vi "Continuous Serial Write and Read 1kHz.vi"() -> ()   [LabVIEW 2017]
doc: "This example performs writes and reads on a serial port, as directed by the user. You can press the Write and Read buttons, and change the Read Count, while the example is running.\n\nThe parameters set for the serial port must match the parameters of the connected instrument or device. In this example, the Read Count parameter specifies the number of bytes that the serial port reads. If there were more bytes at the port than the specified number, those bytes would not be read. If there were less bytes at the port than the specified number, you would receive a timeout error.\n\nThis example expands upon the flow control options for XON and XOFF, allowing the user to choose those control characters. Also, the user can enable or disable a termination character. Some devices require a termination character in order to identify the end of command strings. Some devices send a termination character to signify the end of data to be read. This example shows how you can end the Read operation once a termination character is detected in the buffer and/or append a termination character at the end of the Write data."
uses:
  C:/Program Files (x86)/National Instruments/LabVIEW 2017/examples/Instrument IO/Serial/support/Serial - Settings.ctl
  C:/Program Files (x86)/National Instruments/LabVIEW 2017/examples/Instrument IO/Serial/support/Serial - XON-XOFF Characters.ctl
  C:/Program Files (x86)/National Instruments/LabVIEW 2017/examples/Instrument IO/Serial/support/Serial - ASCII Characters.ctl
  <vilib>/Platform/TimedLoop/XDataNode/timing_clust.ctl
  <vilib>/Platform/TimedLoop/XDataNode/nitl_modes.ctl
  <vilib>/Platform/TimedLoop/XDataNode/wakeup.ctl
  <vilib>/Instr/_visa.llb/VISA Configure Serial Port (Instr).vi
  <vilib>/platform/TimedLoop/XDataNode/XDataNode.xnode
  <vilib>/Platform/TimedLoop/XDataNode/XDNodeRunTimeDep.lvlib
panel:
  in  "Termination Character":u8=10 format="%.0x"
  in  "End Write on Termination Character?":bool=TRUE
  in  "Stop":bool
  in  "Read Count":u32=1000
  out "Response":string="\r\n\r\n\r\n\r\n0.01 0.01 0.01 0.00\r\n0.00 0.00 0.01 0.00\r\n0.00 0.01 0.00 0.00\r\n0.01 0.00 0.01 0.00\r\n0.00 0.01 0.00 0.00\r\n0.01 0.00 0.00 0.00\r\n0.01 0.01 0.01 0.00\r\n0.01 -0.00 -0.00 0.00\r\n0.01 0.01 0.01 0.00\r\n0.01 0.01 0.01 0.00\r\n0.01 0.00 -0.00 0.00\r\n0.00 0.01 0.01 0.00\r\n0.01 0.01 0.00 0.00\r\n0.01 0.01 0.01 0.00\r\n0.00 0.00 0.00 0.00\r\n0.01 0.01 0.01 0.00\r\n0.01 0.00 0.00 0.00\r\n0.00 0.01 0.01 0.00\r\n0.01 0.01 0.01 0.00\r\n0.01 0.01 0.01 0.00\r\n0.01 0.01 0.01 0.00\r\n0.01 0.00 0.01 0.00\r\n0.01 0.00 0.01 0.00\r\n0.01 0.00 0.01 0.00\r\n0.01 0.01 0.01 0.00\r\n0.01 0.00 0.00 0.00\r\n0.00 0.01 0.01 0.00\r\n-0.00 0.01 0.01 0.00\r\n0.00 0.00 0.01 0.00\r\n0.01 0.01 0.01 0.00\r\n0.00 0.01 0.01 0.00\r\n0.01 0.01 0.01 0.00\r\n0.00 0.01 0.01 0.00\r\n0.00 0.01 0.01 0.00\r\n0.01 0.00 0.01 0.00\r\n0.01 0.00 0.00 0.00\r\n0.01 0.01 0.01 0.00\r\n0.00 0.01 0.00 0.00\r\n0.01 0.01 0.01 0.00\r\n0.00 0.01 0.00 0.00\r\n0.01 0.01 0.01 0.00\r\n0.01 0.01 0.01 0.00\r\n0.00 0.01 0.01 0.00\r\n0.01 0.00 0.01 0.00\r\n0.01 0.01 0.01 0.00\r\n0.01 0.01 0.01 0.00\r\n0.00 0.00 0.01 0.00\r\n0.00 -0.00 0.00 0.00\r\n0.01 0.01 0.00 0.00\r\n0.01 0.01 0.01 0.00\r\n0.01 0.00 0.00 0.00\r\n0.01 0.01 0.01 0.00\r\n0.01 0.01 0.00 0.00\r\n0.01 0.01 0.00 0.00\r\n0.01 0.01 0.01 0.00\r\n0.01 0.00 0.01 0.00\r\n0.00 0.01 0.01 0.00\r\n0.01 0.01 0.01 0.00\r\n0.00 0.01 0.01 0.00\r\n0.01 0.00 0.01 0.00\r\n0.01 0.00 0.01 0.00\r\n0.01 0.01 0.01 0.00\r\n0.00 0.01 0.01 0.00\r\n0.01 0.00 0.01 0.00\r\n0.00 0.01 0.00 0.00\r\n0.01 0.01 0.01 0.00\r\n0.00 0.00 0.00 0.00\r\n0.00 0.01 0.00 0.00\r\n0.01 0.00 0.01 0.00\r\n0.01 0.01 0.00 0.00\r\n0.00 0.01 0.00 0.00\r\n0.01 0.01 0.00 0.00\r\n0.01 0.01 0.01 0.00\r\n0.01 0.01 0.01 0.00\r\n0.01 0.01 0.01 0.00\r\n0.01 0.01 0.00 0.00\r\n0.01 0.01 0.01 0.00\r\n0.01 0.00 0.01 0.00\r\n0.00 0.01 0.01 0.00\r\n-0.00 0.01 0.01 0.00\r\n0.00 0.01 0.01 0.00\r\n0.00 -0.00 0.00 0.00\r\n0.01 0.01 0.01 0.00\r\n0.01 0.01 0.00 0.00\r\n0.01 0.01 0.01 0.00\r\n0.00 0.01 0.01 0.00\r\n0.01 0.00 0.01 0.00\r\n0.01 0.00 0.00 0.00\r\n0.01 0.01 0.01 0.00\r\n0.01 0.01 0.01 0.00\r\n0.00 0.01 0.00 0.00\r\n0.01 0.01 0.01 0.00\r\n0.01 0.01 0.00 0.00\r\n0.01 0.00 -0.00 0.00\r\n0.01 0.01 0.01 0.00\r\n0.00 0.00 0.01 0.00\r\n0.00 0.00 0.00 0.00\r\n0.01 0.01 0.01 0.00\r\n0.01 0.01 0.01 0.00\r\n0.01 0.01 0.01 0.00\r\n0.01 0.01 0.01 0.00\r\n0.01 0.01 0.01 0.00\r\n0.01 0.01 0.01 0.00\r\n0.01 0.01 0.01 0.00\r\n0.01 0.01 0.01 0.00\r\n0.01 0.01 0.01 0.00\r\n0.00 0.01 0.01 0.00\r\n0.01 0.01 0.00 0.00\r\n0.01 0.01 0.00 0.00\r\n0.00 0.01 0.01 0.00\r\n0.01 0.01 0.00 0.00\r\n0.01 0.01 0.01 0.00\r\n0.00 0.01 0.01 0.00\r\n0.01 0.02 0.01 0.00\r\n0.01 0.01 0.01 0.00\r\n0.01 0.00 0.00 0.00\r\n0.00 0.01 0.01 0.00\r\n0.01 0.02 0.01 0.00\r\n0.01 0.01 0.01 0.00\r\n0.01 0.01 0.01 0.00\r\n0.01 0.00 0.01 0.00\r\n0.01 0.01 0.01 0.00\r\n0.01 0.01 0.01 0.00\r\n0.00 0.00 0.01 0.00\r\n0.01 0.00 0.00 0.00\r\n0.00 0.00 0.01 0.00\r\n0.01 0.01 0.01 0.00\r\n0.01 0.01 0.00 0.00\r\n0.00 0.01 0.01 0.00\r\n0.01 0.00 0.01 0.00\r\n0.01 0.00 0.01 0.00\r\n0.01 0.01 0.01 0.00\r\n0.01 0.01 0.01 0.00\r\n0.00 0.00 0.00 0.00\r\n0.01 0.01 0.01 0.00\r\n0.00 0.01 0.01 0.00\r\n0.01 0.00 0.00 0.00\r\n0.00 0.01 0.00 0.00\r\n0.01 0.01 0.02 0.00\r\n0.00 0.01 0.01 0.00\r\n0.00 0.01 0.01 0.00\r\n0.01 0.01 0.01 0.00\r\n0.01 0.00 0.01 0.00\r\n0.01 0.01 0.01 0.00\r\n0.01 0.01 0.01 0.00\r\n0.01 0.01 0.01 0.00\r\n0.01 0.01 0.01 0.00\r\n0.01 0.01 0.01 0.00\r\n0.00 0.01 0.01 0.00\r\n0.00 0.01 0.01 0.00\r\n0.01 0.01 0.01 0.00\r\n0.01 0.01 0.01 0.00\r\n0.01 0.00 0.01 0.00\r\n0.01 0.01 0.01 0.00\r\n0.01 0.01 0.01 0.00\r\n0.01 0.01 0.01 0.00\r\n0.01 0.01 0.01 0.00\r\n0.01 0.01 0.02 0.00\r\n0.01 0.01 0.01 0.00\r\n0.00 0.00 0.01 0.00\r\n0.01 0.01 0.01 0.00\r\n0.00 0.01 0.01 0.00\r\n0.01 0.01 0.01 0.00\r\n0.00 0.01 0.01 0.00\r\n0.00 0.01 0.01 0.00\r\n0.00 0.01 0.01 0.00\r\n0.01 0.00 0.01 0.00\r\n0.01 0.01 0.01 0.00\r\n0.01 0.01 0.01 0.00\r\n0.01 0.00 0.01 0.00\r\n0.01 0.01 0.01 0.00\r\n0.01 0.01 0.01 0.00\r\n0.01 0.01 0.01 0.00\r\n0.01 0.00 0.00 0.00\r\n0.01 0.01 0.01 0.00\r\n0.01 0.01 0.01 0.00\r\n0.01 -0.00 0.00 0.00\r\n0.00 0.01 0.01 0.00\r\n0.01 0.01 0.01 0.00\r\n0.01 0.01 0.00 0.00\r\n0.00 0.00 0.00 0.00\r\n0.01 0.00 0.00 0.00\r\n0.01 0.00 0.00 0.00\r\n0.00 0.01 0.01 0.00\r\n0.01 0.01 0.01 0.00\r\n0.01 0.01 0.01 0.00\r\n0.01 0.01 0.01 0.00\r\n0.00 0.01 0.01 0.00\r\n0.01 0.00 0.00 0.00\r\n0.01 0.01 0.00 0.00\r\n0.01 0.01 0.01 0.00\r\n0.00 0.00 0.00 0.00\r\n0.01 0.01 0.01 0.00\r\n0.01 0.01 0.01 0.00\r\n0.01 0.02 0.01 0.00\r\n0.01 0.00 0.01 0.00\r\n0.00 0.01 0.01 0.00\r\n0.00 0.00 0.00 0.00\r\n0.01 0.01 0.01 0.00\r\n0.01 0.00 0.00 0.00\r\n0.01 0.01 0.01 0.00\r\n0.01 -0.00 -0.00 0.00\r\n0.00 0.01 0.01 0.00\r\n0.01 0.01 0.01 0.00\r\n0.00 0.01 0.01 0.00\r\n0.01 0.01 0.01 0.00\r\n0.01 0.01 0.01 0.00\r\n0.00 0.01 0.01 0.00\r\n0.01 0.01 0.01 0.00\r\n0.01 0.01 0.01 0.00\r\n0.01 0.01 0.00 0.00\r\n0.00 0.00 0.00 0.00\r\n0.01 0.01 0.01 0.00\r\n0.01 0.00 0.01 0.00\r\n0.01 0.01 0.01 0.00\r\n0.01 0.01 0.01 0.00\r\n0.01 0.00 0.00 0.00\r\n0.00 0.01 0.00 0.00\r\n0.01 0.01 0.01 0.00\r\n0.01 0.00 0.01 0.00\r\n0.01 0.01 0.01 0.00\r\n0.00 0.01 0.01 0.00\r\n0.01 0.00 0.01 0.00\r\n0.01 0.01 0.00 0.00\r\n0.01 0.00 0.01 0.00\r\n0.01 0.01 0.00 0.00\r\n0.01 0.01 0.01 0.00\r\n0.01 0.01 0.00 0.00\r\n0.01 0.00 0.01 0.00\r\n0.00 0.01 0.01 0.00\r\n0.01 0.01 0.01 0.00\r\n0.01 0.00 0.00 0.00\r\n0.00 0.01 0.00 0.00\r\n-0.00 0.01 0.00 0.00\r\n0.01 0.00 0.00 0.00\r\n0.01 0.01 0.01 0.00\r\n0.01 0.01 0.01 0.00\r\n0.01 0.01 0.01 0.00\r\n0.01 0.01 0.01 0.00\r\n0.01 0.01 0.01 0.00\r\n0.01 0.01 0.01 0.00\r\n0.01 0.01 0.01 0.00\r\n0.00 0.01 0.00 0.00\r\n0.01 0.00 0.01 0.00\r\n0.01 0.01 0.00 0.00\r\n0.00 0.00 0.01 0.00\r\n0.01 0.01 0.00 0.00\r\n0.01 0.00 0.01 0.00\r\n0.00 0.01 0.01 0.00\r\n0.01 0.00 0.00 0.00\r\n0.01 0.00 0.01 0.00\r\n0.01 0.01 0.01 0.00\r\n0.01 0.01 0.01 0.00\r\n0.01 0.00 0.00 0.00\r\n0.01 0.01 0.01 0.00\r\n0.01 -0.00 0.01 0.00\r\n0.01 0.00 0.01 0.00\r\n0.00 0.01 0.01 0.00\r\n0.01 0.01 0.01 0.00\r\n0.01 0.01 0.01 0.00\r\n0.00 0.01 0.01 0.00\r\n0.00 0.00 0.00 0.00\r\n0.01 0.01 0.01 0.00\r\n0.00 0.01 0.01 0.00\r\n0.01 0.01 0.01 0.00\r\n0.01 0.00 0.00 0.00\r\n0.00 0.01 0.01 0.00\r\n0.01 0.01 0.01 0.00\r\n0.01 0.01 0.00 0.00\r\n-0.00 0.01 0.00 0.00\r\n0.01 0.01 0.01 0.00\r\n0.01 0.01 0.01 0.00\r\n0.01 0.01 0.01 0.00\r\n0.01 0.01 0.01 0.00\r\n0.01 0.00 0.01 0.00\r\n0.01 0.01 0.01 0.00\r\n0.01 0.01 0.00 0.00\r\n0.01 0.01 0.01 0.00\r\n0.00 0.01 0.01 0.00\r\n0.00 0.01 0.01 0.00\r\n0.01 0.00 0.01 0.00\r\n0.01 0.00 -0.00 0.00\r\n0.00 0.00 0.01 0.00\r\n0.00 0.00 0.01 0.00\r\n0.00 0.00 0.01 0.00\r\n0.01 0.01 0.01 0.00\r\n0.01 0.01 0.01 0.00\r\n-0.00 0.00 -0.00 0.00\r\n0.01 0.01 0.01 0.00\r\n0.01 0.00 0.00 0.00\r\n-0.00 0.00 0.00 0.00\r\n0.01 0.01 0.01 0.00\r\n0.01 0.01 0.00 0.00\r\n0.01 0.01 0.01 0.00\r\n0.00 0.01 0.01 0.00\r\n0.00 0.00 0.01 0.00\r\n0.00 0.01 0.01 0.00\r\n0.01 0.01 0.01 0.00\r\n0.01 0.01 -0.00 0.00\r\n0.00 0.01 0.01 0.00\r\n0.01 0.01 0.01 0.00\r\n0.01 0.01 0.01 0.00\r\n0.01 -0.00 0.00 0.00\r\n0.01 0.01 0.01 0.00\r\n0.00 0.01 0.01 0.00\r\n0.01 0.01 0.01 0.00\r\n0.00 0.01 0.01 0.00\r\n0.01 0.00 0.01 0.00\r\n0.01 0.01 0.01 0.00\r\n0.00 0.01 0.00 0.00\r\n0.01 0.01 0.01 0.00\r\n0.01 0.00 0.00 0.00\r\n0.00 0.01 0.01 0.00\r\n0.01 0.01 0.01 0.00\r\n0.00 0.00 0.00 0.00\r\n0.01 0.01 0.01 0.00\r\n0.01 0.01 0.01 0.00\r\n0.01 0.01 0.01 0.00\r\n0.01 0.01 0.01 0.00\r\n0.01 0.00 0.01 0.00\r\n0.00 0.01 0.00 0.00\r\n0.00 0.01 0.01 0.00\r\n0.01 0.01 0.01 0.00\r\n0.01 0.00 0.01 0.00\r\n-0.00 0.01 0.00 0.00\r\n0.01 0.01 0.01 0.00\r\n0.01 0.00 0.01 0.00\r\n0.01 0.01 0.01 0.00\r\n0.01 0.01 0.01 0.00\r\n0.01 0.01 0.01 0.00\r\n0.01 0.00 0.00 0.00\r\n0.00 0.01 0.00 0.00\r\n0.02 0.00 0.01 0.00\r\n0.00 0.00 0.00 0.00\r\n0.01 0.00 0.00 0.00\r\n0.00 0.00 0.00 0.00\r\n0.01 0.00 0.01 0.00\r\n0.00 0.01 0.01 0.00\r\n0.01 0.01 0.01 0.00\r\n-0.00 0.01 0.00 0.00\r\n0.01 0.01 0.00 0.00\r\n0.01 0.00 0.01 0.00\r\n0.00 0.00 0.00 0.00\r\n0.01 0.01 0.01 0.00\r\n0.01 0.00 0.00 0.00\r\n0.01 0.01 0.01 0.00\r\n0.01 0.01 0.01 0.00\r\n0.00 0.01 0.01 0.00\r\n0.01 0.01 0.01 0.00\r\n0.01 0.01 0.01 0.00\r\n0.00 0.00 0.01 0.00\r\n0.01 0.01 0.01 0.00\r\n0.01 0.01 0.01 0.00\r\n0.01 0.01 0.01 0.00\r\n0.01 0.01 0.01 0.00\r\n0.01 0.01 0.01 0.00\r\n0.01 0.01 0.01 0.00\r\n0.01 0.01 0.01 0.00\r\n0.00 0.00 0.01 0.00\r\n0.01 0.01 0.01 0.00\r\n0.01 0.01 0.01 0.00\r\n0.01 0.01 0.01 0.00\r\n0.01 0.01 0.01 0.00\r\n0.01 0.01 0.01 0.00\r\n0.01 0.01 0.01 0.00\r\n0.01 0.01 0.01 0.00\r\n0.01 0.01 0.01 0.00\r\n0.01 0.01 0.00 0.00\r\n0.01 0.01 0.01 0.00\r\n0.01 0.01 0.01 0.00\r\n0.01 0.00 0.01 0.00\r\n0.00 0.00 0.00 0.00\r\n0.01 0.00 0.01 0.00\r\n0.01 0.01 0.01 0.00\r\n0.01 0.01 0.01 0.00\r\n0.01 0.01 0.01 0.00\r\n0.01 0.01 0.01 0.00\r\n0.01 0.00 0.01 0.00\r\n0.01 0.01 0.01 0.00\r\n0.01 0.01 0.01 0.00\r\n0.01 0.00 0.01 0.00\r\n0.00 0.01 0.01 0.00\r\n0.01 0.01 0.01 0.00\r\n0.01 0.01 0.01 0.00\r\n0.01 0.00 0.01 0.00\r\n0.01 0.01 0.00 0.00\r\n0.01 0.00 0.01 0.00\r\n0.01 0.01 0.01 0.00\r\n0.00 0.01 0.01 0.00\r\n0.01 0.01 0.00 0.00\r\n0.00 0.01 0.01 0.00\r\n0.01 0.00 0.01 0.00\r\n0.01 0.00 0.00 0.00\r\n0.01 0.00 0.01 0.00\r\n0.01 0.01 0.00 0.00\r\n0.01 0.01 0.01 0.00\r\n0.01 0.01 0.00 0.00\r\n0.01 0.00 0.01 0.00\r\n0.01 0.01 0.01 0.00\r\n0.01 0.01 0.01 0.00\r\n0.01 -0.00 0.01 0.00\r\n0.01 0.01 0.01 0.00\r\n0.01 0.00 0.01 0.00\r\n0.01 0.01 0.01 0.00\r\n0.00 0.01 0.01 0.00\r\n0.01 0.01 0.01 0.00\r\n0.00 0.00 0.00 0.00\r\n0.01 0.01 0.00 0.00\r\n0.01 0.01 0.02 0.00\r\n0.01 0.00 0.01 0.00\r\n0.00 0.00 0.00 0.00\r\n0.01 0.01 0.01 0.00\r\n0.01 0.01 0.01 0.00\r\n0.01 0.01 0.01 0.00\r\n0.01 0.01 0.01 0.00\r\n0.00 0.00 0.01 0.00\r\n0.01 0.01 0.01 0.00\r\n0.01 0.01 0.01 0.00\r\n0.00 0.01 0.01 0.00\r\n0.01 0.00 0.01 0.00\r\n0.01 0.01 0.01 0.00\r\n0.01 0.00 0.00 0.00\r\n0.00 0.01 0.01 0.00\r\n0.01 0.01 0.01 0.00\r\n0.01 0.01 0.01 0.00\r\n0.01 0.01 0.01 0.00\r\n0.01 0.01 0.00 0.00\r\n0.01 0.01 0.00 0.00\r\n0.01 0.00 0.01 0.00\r\n0.01 0.01 0.01 0.00\r\n0.01 0.00 0.01 0.00\r\n0.00 0.01 0.01 0.00\r\n0.00 0.01 0.01 0.00\r\n0.01 0.01 0.01 0.00\r\n0.00 0.01 0.01 0.00\r\n0.01 0.01 0.01 0.00\r\n0.01 0.01 0.01 0.00\r\n0.01 0.01 0.01 0.00\r\n0.01 0.00 0.00 0.00\r\n0.01 0.00 0.01 0.00\r\n0.01 0.00 0.01 0.00\r\n0.01 0.01 0.01 0.00\r\n-0.00 0.01 0.00 0.00\r\n0.01 0.00 0.01 0.00\r\n0.01 0.01 0.01 0.00\r\n0.01 0.01 0.00 0.00\r\n0.01 0.00 0.01 0.00\r\n0.01 0.01 0.01 0.00\r\n0.00 0.01 0.01 0.00\r\n0.01 0.01 0.00 0.00\r\n0.00 0.01 0.01 0.00\r\n0.01 0.01 0.01 0.00\r\n0.01 0.00 0.01 0.00\r\n0.00 0.01 0.01 0.00\r\n0.01 0.01 0.00 0.00\r\n0.01 0.01 0.00 0.00\r\n0.00 0.01 0.01 0.00\r\n0.00 0.01 0.01 0.00\r\n0.01 0.01 0.01 0.00\r\n0.01 0.01 0.01 0.00\r\n0.01 0.01 0.01 0.00\r\n0.01 0.01 0.01 0.00\r\n0.00 0.01 0.01 0.00\r\n0.01 0.01 0.00 0.00\r\n0.01 0.00 0.01 0.00\r\n0.01 0.01 0.01 0.00\r\n0.00 0.01 0.01 0.00\r\n0.01 0.02 0.01 0.00\r\n0.01 0.00 0.01 0.00\r\n0.01 0.01 0.01 0.00\r\n0.01 0.01 0.01 0.00\r\n0.01 0.01 0.01 0.00\r\n0.01 0.01 0.01 0.00\r\n0.01 0.01 0.01 0.00\r\n0.01 0.01 0.01 0.00\r\n-0.00 0.01 0.00 0.00\r\n0.01 0.01 0.01 0.00\r\n0.01 0.01 0.01 0.00\r\n0.01 0.01 0.01 0.00\r\n0.01 0.01 0.01 0.00\r\n0.01 0.01 0.01 0.00\r\n0.00 0.00 0.00 0.00\r\n0.01 0.00 0.00 0.00\r\n0.01 0.01 0.01 0.00\r\n0.00 0.01 0.01 0.00\r\n0.01 0.01 0.01 0.00\r\n0.01 0.00 0.01 0.00\r\n-0.00 0.01 0.01 0.00\r\n0.00 0.01 0.01 0.00\r\n0.01 0.00 0.00 0.00\r\n0.00 0.01 0.00 0.00\r\n0.01 0.01 0.01 0.00\r\n0.00 0.00 0.00 0.00\r\n0.01 0.01 0.01 0.00\r\n0.01 0.01 0.02 0.00\r\n0.00 0.01 0.01 0.00\r\n0.00 0.00 0.00 0.00\r\n0.01 0.00 0.01 0.00\r\n0.01 0.00 0.01 0.00\r\n0.00 0.01 0.01 0.00\r\n0.01 0.01 0.01 0.00\r\n0.01 0.00 0.00 0.00\r\n0.01 0.01 0.01 0.00\r\n0.01 0.01 0.01 0.00\r\n0.01 0.00 0.00 0.00\r\n0.01 -0.00 0.00 0.00\r\n0.00 0.01 0.00 0.00\r\n0.01 0.01 0.01 0.00\r\n0.01 0.01 0.01 0.00\r\n0.00 0.00 0.00 0.00\r\n0.01 0.00 0.01 0.00\r\n0.01 0.01 0.01 0.00\r\n0.01 0.00 0.00 0.00\r\n0.01 0.01 0.01 0.00\r\n0.00 0.01 0.01 0.00\r\n0.01 0.01 0.01 0.00\r\n0.01 0.01 0.01 0.00\r\n0.01 0.01 0.01 0.00\r\n0.01 0.01 0.01 0.00\r\n0.01 0.00 0.01 0.00\r\n0.01 0.00 0.01 0.00\r\n0.01 0.00 0.01 0.00\r\n0.01 -0.00 0.01 0.00\r\n0.01 0.00 0.00 0.00\r\n0.01 0.01 0.01 0.00\r\n0.00 0.01 0.01 0.00\r\n0.01 0.01 0.01 0.00\r\n0.00 0.01 0.00 0.00\r\n0.00 0.00 0.00 0.00\r\n0.01 0.01 0.01 0.00\r\n0.01 0.01 0.01 0.00\r\n0.01 0.01 0.01 0.00\r\n0.00 0.00 0.00 0.00\r\n0.01 0.01 -0.00 0.00\r\n0.00 0.01 0.01 0.00\r\n0.00 0.01 0.01 0.00\r\n0.01 0.01 0.01 0.00\r\n0.01 0.00 0.01 0.00\r\n0.01 0.01 0.01 0.00\r\n0.00 0.00 -0.00 0.00\r\n0.00 0.01 0.01 0.00\r\n0.01 0.00 0.00 0.00\r\n0.01 0.00 0.01 0.00\r\n0.01 0.01 0.00 0.00\r\n0.01 0.01 0.01 0.00\r\n0.00 0.01 0.01 0.00\r\n0.00 0.01 0.00 0.00\r\n0.00 0.00 0.01 0.00\r\n0.01 0.00 -0.00 0.00\r\n0.01 0.01 0.01 0.00\r\n0.01 0.01 0.01 0.00\r\n0.00 0.00 0.01 0.00\r\n0.00 0.01 0.01 0.00\r\n0.00 0.00 0.01 0.00\r\n0.01 0.01 0.01 0.00\r\n0.01 0.01 0.00 0.00\r\n0.01 0.01 0.01 0.00\r\n0.01 0.00 0.01 0.00\r\n0.00 0.00 0.01 0.00\r\n0.01 0.01 0.01 0.00\r\n0.02 0.01 0.01 0.00\r\n0.01 0.01 0.01 0.00\r\n0.01 0.00 0.01 0.00\r\n0.01 0.00 0.01 0.00\r\n0.01 0.00 0.01 0.00\r\n0.00 0.00 0.00 0.00\r\n0.01 0.00 0.01 0.00\r\n0.01 0.01 0.01 0.00\r\n0.01 0.00 0.00 0.00\r\n0.01 0.01 0.01 0.00\r\n0.01 0.01 0.01 0.00\r\n0.00 0.01 0.01 0.00\r\n0.01 0.01 0.01 0.00\r\n-0.00 0.00 -0.00 0.00\r\n0.01 0.00 0.01 0.00\r\n0.00 0.00 0.00 0.00\r\n0.01 0.01 0.01 0.00\r\n0.00 0.01 0.01 0.00\r\n0.00 0.00 0.00 0.00\r\n0.00 0.01 0.01 0.00\r\n0.00 0.01 0.01 0.00\r\n0.00 0.01 0.01 0.00\r\n0.01 0.01 0.00 0.00\r\n0.01 0.01 0.00 0.00\r\n0.01 0.00 0.00 0.00\r\n0.01 0.01 0.01 0.00\r\n0.01 0.01 0.01 0.00\r\n0.00 0.01 0.01 0.00\r\n0.01 0.01 0.01 0.00\r\n0.01 0.01 0.01 0.00\r\n0.01 0.01 0.01 0.00\r\n0.01 0.00 0.01 0.00\r\n0.01 0.01 0.00 0.00\r\n0.01 0.00 0.01 0.00\r\n0.01 0.00 0.00 0.00\r\n0.01 0.01 0.01 0.00\r\n0.00 0.01 0.00 0.00\r\n0.01 0.01 0.01 0.00\r\n0.00 0.01 0.01 0.00\r\n0.01 0.01 0.01 0.00\r\n0.00 0.01 0.01 0.00\r\n0.01 0.00 0.00 0.00\r\n0.01 0.01 0.01 0.00\r\n0.01 -0.00 -0.00 0.00\r\n0.01 0.01 0.01 0.00\r\n0.01 0.01 0.01 0.00\r\n0.01 0.00 0.01 0.00\r\n0.01 0.01 0.00 0.00\r\n0.01 0.01 0.01 0.00\r\n0.01 0.01 0.01 0.00\r\n0.01 0.00 0.00 0.00\r\n0.00 0.00 0.00 0.00\r\n0.01 0.01 0.01 0.00\r\n0.00 0.01 0.00 0.00\r\n0.01 0.01 0.01 0.00\r\n0.01 0.01 0.01 0.00\r\n0.00 0.01 0.00 0.00\r\n0.01 0.00 0.01 0.00\r\n0.01 0.01 0.01 0.00\r\n0.00 0.01 0.01 0.00\r\n0.01 0.00 0.00 0.00\r\n0.01 0.00 0.01 0.00\r\n0.01 0.01 0.01 0.00\r\n0.00 0.01 0.01 0.00\r\n0.00 0.01 0.01 0.00\r\n0.00 0.01 0.01 0.00\r\n0.01 0.01 0.01 0.00\r\n0.01 0.01 0.00 0.00\r\n0.00 0.01 0.00 0.00\r\n0.01 0.01 0.00 0.00\r\n0.01 0.01 0.01 0.00\r\n0.01 0.01 0.01 0.00\r\n0.00 0.01 0.01 0.00\r\n0.01 0.01 0.01 0.00\r\n0.01 -0.00 0.00 0.00\r\n0.00 0.01 0.01 0.00\r\n0.01 0.00 0.00 0.00\r\n0.00 0.00 0.00 0.00\r\n0.01 0.01 0.00 0.00\r\n0.01 0.00 0.01 0.00\r\n0.01 0.00 0.00 0.00\r\n0.00 0.01 0.01 0.00\r\n0.01 0.00 0.01 0.00\r\n0.00 0.01 0.01 0.00\r\n0.01 0.01 0.01 0.00\r\n0.00 0.01 0.01 0.00\r\n0.01 0.00 0.00 0.00\r\n0.01 0.01 0.00 0.00\r\n0.01 0.00 0.01 0.00\r\n0.01 0.00 0.01 0.00\r\n0.01 0.01 0.00 0.00\r\n0.01 0.01 0.01 0.00\r\n0.01 0.01 0.01 0.00\r\n0.01 0.01 0.00 0.00\r\n0.00 0.00 0.01 0.00\r\n0.01 0.01 0.01 0.00\r\n0.01 0.00 0.01 0.00\r\n0.01 0.01 0.00 0.00\r\n0.01 0.01 0.00 0.00\r\n0.01 0.01 0.01 0.00\r\n0.00 0.01 0.00 0.00\r\n0.01 0.00 0.01 0.00\r\n0.01 0.01 0.01 0.00\r\n-0.00 0.01 -0.00 0.00\r\n0.01 0.01 0.01 0.00\r\n0.01 0.00 0.01 0.00\r\n0.00 0.00 0.00 0.00\r\n0.01 0.00 0.00 0.00\r\n0.01 0.01 0.00 0.00\r\n0.01 0.02 0.01 0.00\r\n0.01 0.01 0.01 0.00\r\n0.01 0.00 0.01 0.00\r\n0.00 0.01 0.01 0.00\r\n0.01 0.01 0.01 0.00\r\n0.01 0.01 0.01 0.00\r\n0.01 0.01 0.00 0.00\r\n0.01 0.01 0.01 0.00\r\n0.00 0.01 0.00 0.00\r\n0.00 0.01 0.00 0.00\r\n0.01 0.01 0.01 0.00\r\n0.01 0.01 0.01 0.00\r\n0.01 0.00 -0.00 0.00\r\n0.01 0.01 0.01 0.00\r\n0.01 -0.00 0.00 0.00\r\n0.00 0.01 0.01 0.00\r\n0.00 0.01 0.01 0.00\r\n0.01 0.01 0.01 0.00\r\n0.00 0.00 0.01 0.00\r\n0.00 0.00 0.00 0.00\r\n0.01 0.01 0.01 0.00\r\n0.01 0.00 0.00 0.00\r\n0.01 0.01 0.01 0.00\r\n0.01 0.01 0.01 0.00\r\n0.01 0.00 0.01 0.00\r\n0.01 0.01 0.00 0.00\r\n0.01 0.00 0.01 0.00\r\n0.01 0.01 0.01 0.00\r\n0.01 0.01 0.01 0.00\r\n0.01 0.01 0.01 0.00\r\n0.01 0.00 0.00 0.00\r\n0.01 0.01 0.01 0.00\r\n0.01 0.01 0.01 0.00\r\n0.00 0.01 -0.00 0.00\r\n0.01 0.01 0.01 0.00\r\n0.01 0.00 0.01 0.00\r\n0.01 0.01 0.01 0.00\r\n0.01 0.01 0.01 0.00\r\n0.01 0.01 0.01 0.00\r\n0.01 0.01 0.01 0.00\r\n0.01 0.00 0.01 0.00\r\n0.01 0.01 0.01 0.00\r\n0.00 0.01 0.00 0.00\r\n0.01 0.01 0.01 0.00\r\n0.01 0.01 0.01 0.00\r\n0.00 0.00 0.00 0.00\r\n0.01 0.01 0.01 0.00\r\n0.01 0.00 0.01 0.00\r\n0.00 0.01 0.00 0.00\r\n0.01 0.00 0.01 0.00\r\n0.01 0.01 0.01 0.00\r\n0.01 0.00 0.01 0.00\r\n0.01 0.01 0.01 0.00\r\n0.01 0.01 0.01 0.00\r\n0.00 0.01 0.01 0.00\r\n0.01 0.01 0.01 0.00\r\n0.01 0.01 0.01 0.00\r\n0.00 0.01 0.01 0.00\r\n0.01 0.01 0.01 0.00\r\n0.00 0.01 0.01 0.00\r\n0.01 0.01 0.00 0.00\r\n0.01 0.01 0.00 0.00\r\n0.01 0.00 0.00 0.00\r\n0.00 0.01 0.01 0.00\r\n0.01 0.01 0.01 0.00\r\n0.01 0.01 0.01 0.00\r\n0.01 0.01 0.01 0.00\r\n0.01 0.01 0.01 0.00\r\n0.01 0.01 0.01 0.00\r\n0.01 0.01 0.01 0.00\r\n0.00 0.00 0.00 0.00\r\n0.01 0.01 0.01 0.00\r\n0.00 0.00 0.00 0.00\r\n0.01 0.00 0.01 0.00\r\n0.01 0.01 0.00 0.00\r\n0.01 0.01 0.01 0.00\r\n0.01 0.00 0.00 0.00\r\n0.01 0.01 0.01 0.00\r\n0.00 0.01 0.01 0.00\r\n0.00 0.00 0.00 0.00\r\n0.01 0.01 0.00 0.00\r\n0.01 0.01 0.01 0.00\r\n0.01 0.01 0.01 0.00\r\n0.01 0.01 0.01 0.00\r\n0.01 0.00 0.01 0.00\r\n0.01 0.01 0.00 0.00\r\n0.01 0.01 0.01 0.00\r\n0.01 0.00 0.01 0.00\r\n0.01 0.01 0.00 0.00\r\n0.01 0.01 0.00 0.00\r\n0.01 0.01 0.01 0.00\r\n0.01 0.01 0.01 0.00\r\n0.00 0.01 0.00 0.00\r\n0.01 0.01 0.01 0.00\r\n0.00 0.01 0.01 0.00\r\n0.01 0.01 0.01 0.00\r\n0.00 0.01 0.01 0.00\r\n0.01 -0.00 0.01 0.00\r\n0.00 0.01 0.01 0.00\r\n0.01 0.01 0.01 0.00\r\n0.01 0.01 0.01 0.00\r\n-0.00 0.00 0.00 0.00\r\n0.01 0.01 0.01 0.00\r\n0.00 0.01 0.01 0.00\r\n0.01 0.01 0.01 0.00\r\n0.00 0.01 0.01 0.00\r\n0.02 0.01 0.01 0.00\r\n0.01 0.01 0.01 0.00\r\n0.01 0.01 0.01 0.00\r\n0.00 0.00 0.00 0.00\r\n0.00 0.00 0.00 0.00\r\n0.01 0.01 0.01 0.00\r\n0.01 0.01 0.01 0.00\r\n0.01 0.01 0.01 0.00\r\n0.01 0.01 0.01 0.00\r\n0.01 0.01 0.01 0.00\r\n0.00 0.01 0.01 0.00\r\n0.01 0.01 0.01 0.00\r\n0.02 0.01 0.01 0.00\r\n0.01 0.01 0.01 0.00\r\n0.00 0.02 0.01 0.00\r\n0.00 0.01 0.00 0.00\r\n0.00 0.01 0.00 0.00\r\n0.01 0.01 0.00 0.00\r\n0.01 0.00 0.01 0.00\r\n0.01 0.00 0.01 0.00\r\n0.00 0.01 0.01 0.00\r\n0.01 0.01 0.01 0.00\r\n0.01 0.00 0.01 0.00\r\n0.00 0.01 0.01 0.00\r\n0.01 0.01 0.01 0.00\r\n0.01 0.01 0.00 0.00\r\n0.01 0.00 0.01 0.00\r\n0.00 0.01 0.01 0.00\r\n0.00 0.01 -0.00 0.00\r\n0.01 0.01 0.01 0.00\r\n0.01 0.00 0.01 0.00\r\n0.00 0.00 0.00 0.00\r\n0.00 0.01 0.00 0.00\r\n0.01 0.01 0.01 0.00\r\n0.00 0.00 0.00 0.00\r\n0.00 0.01 0.01 0.00\r\n0.01 0.00 0.01 0.00\r\n0.01 0.00 0.01 0.00\r\n0.01 0.01 0.00 0.00\r\n0.01 0.01 0.02 0.00\r\n0.01 0.01 0.00 0.00\r\n0.00 0.01 0.01 0.00\r\n0.00 0.01 0.00 0.00\r\n0.01 0.00 0.00 0.00\r\n0.01 0.01 0.01 0.00\r\n0.01 0.01 0.01 0.00\r\n0.01 0.00 0.01 0.00\r\n0.00 0.01 0.01 0.00\r\n0.01 0.01 0.01 0.00\r\n0.01 0.01 0.01 0.00\r\n0.01 0.01 0.00 0.00\r\n0.01 0.01 0.01 0.00\r\n0.00 0.01 0.01 0.00\r\n0.01 0.01 0.01 0.00\r\n0.01 0.01 0.01 0.00\r\n0.01 0.01 0.01 0.00\r\n0.01 0.00 0.00 0.00\r\n0.01 0.01 0.01 0.00\r\n0.01 0.00 0.00 0.00\r\n0.01 0.00 0.01 0.00\r\n0.01 0.00 0.00 0.00\r\n0.01 0.01 0.01 0.00\r\n0.00 0.01 0.00 0.00\r\n0.01 0.01 0.01 0.00\r\n0.01 0.01 0.01 0.00\r\n0.00 0.01 0.01 0.00\r\n0.01 0.00 0.01 0.00\r\n0.01 0.01 0.01 0.00\r\n0.01 0.01 0.01 0.00\r\n0.01 0.01 0.01 0.00\r\n0.01 0.01 0.01 0.00\r\n0.01 0.00 0.01 0.00\r\n0.00 0.00 0.00 0.00\r\n0.00 0.01 0.00 0.00\r\n0.01 0.01 -0.00 0.00\r\n0.00 0.01 0.01 0.00\r\n0.01 0.01 0.01 0.00\r\n0.01 0.00 0.01 0.00\r\n0.01 0.01 0.01 0.00\r\n0.01 0.01 0.01 0.00\r\n0.01 0.00 0.01 0.00\r\n0.00 0.01 0.01 0.00\r\n0.01 0.01 0.01 0.00\r\n0.01 0.00 0.00 0.00\r\n0.00 0.00 0.00 0.00\r\n0.01 0.01 0.01 0.00\r\n0.00 0.01 0.01 0.00\r\n0.00 0.01 0.00 0.00\r\n0.01 0.01 0.01 0.00\r\n0.01 0.01 0.01 0.00\r\n0.00 0.01 0.00 0.00\r\n0.01 0.01 0.01 0.00\r\n0.01 0.01 0.01 0.00\r\n0.01 0.01 0.00 0.00\r\n0.01 0.01 0.01 0.00\r\n0.01 0.00 0.00 0.00\r\n0.00 0.00 0.00 0.00\r\n0.01 0.00 0.00 0.00\r\n0.01 0.01 0.01 0.00\r\n0.01 0.00 0.00 0.00\r\n0.01 0.00 0.00 0.00\r\n0.01 0.01 0.01 0.00\r\n0.00 0.01 0.00 0.00\r\n0.01 0.01 0.01 0.00\r\n0.01 0.01 0.00 0.00\r\n-0.00 0.00 0.00 0.00\r\n0.00 0.01 0.01 0.00\r\n0.01 0.01 0.01 0.00\r\n0.01 0.01 0.00 0.00\r\n0.01 0.01 0.01 0.00\r\n0.02 0.01 0.01 0.00\r\n0.00 0.01 0.00 0.00\r\n0.01 0.01 0.01 0.00\r\n0.00 0.01 0.01 0.00\r\n0.01 -0.00 0.01 0.00\r\n0.00 0.01 0.00 0.00\r\n0.01 0.01 0.01 0.00\r\n0.00 0.00 -0.00 0.00\r\n0.01 0.01 0.01 0.00\r\n0.01 0.01 0.00 0.00\r\n0.00 0.01 0.01 0.00\r\n0.00 0.01 0.00 0.00\r\n0.00 0.00 0.01 0.00\r\n0.00 0.01 0.00 0.00\r\n0.01 0.00 0.01 0.00\r\n0.01 0.01 0.01 0.00\r\n0.01 0.01 0.01 0.00\r\n0.01 0.01 0.01 0.00\r\n0.01 0.00 0.01 0.00\r\n0.00 0.01 0.01 0.00\r\n0.01 0.01 0.01 0.00\r\n0.01 0.00 0.00 0.00\r\n0.01 0.00 0.01 0.00\r\n-0.00 0.01 0.01 0.00\r\n0.01 0.01 0.01 0.00\r\n0.01 0.00 0.01 0.00\r\n0.01 0.01 0.01 0.00\r\n0.01 0.01 0.01 0.00\r\n0.02 -0.00 0.00 0.00\r\n0.01 0.01 0.00 0.00\r\n0.01 0.00 0.01 0.00\r\n0.01 0.01 0.01 0.00\r\n0.00 0.01 0.01 0.00\r\n0.01 0.01 0.01 0.00\r\n0.01 0.01 0.01 0.00\r\n0.01 0.00 0.00 0.00\r\n0.01 0.00 0.01 0.00\r\n0.02 0.01 0.01 0.00\r\n0.00 0.01 -0.00 0.00\r\n0.01 0.00 0.00 0.00\r\n0.01 0.01 0.00 0.00\r\n0.01 0.01 0.01 0.00\r\n0.00 0.01 0.01 0.00\r\n0.01 0.01 0.01 0.00\r\n0.00 0.01 0.01 0.00\r\n0.00 0.01 0.01 0.00\r\n0.01 0.01 0.01 0.00\r\n0.01 0.00 0.00 0.00\r\n0.01 0.01 0.01 0.00\r\n0.01 0.01 0.01 0.00\r\n0.00 0.01 0.01 0.00\r\n0.01 0.01 0.01 0.00\r\n0.01 0.01 0.01 0.00\r\n0.00 0.00 0.00 0.00\r\n0.01 0.01 0.01 0.00\r\n0.01 0.01 0.00 0.00\r\n0.01 0.00 0.01 0.00\r\n0.01 0.01 0.01 0.00\r\n0.01 0.01 0.01 0.00\r\n0.01 0.01 0.00 0.00\r\n0.01 0.01 0.01 0.00\r\n0.01 0.01 0.01 0.00\r\n0.00 0.01 0.00 0.00\r\n0.01 0.00 0.01 0.00\r\n0.01 0.01 0.01 0.00\r\n0.00 0.01 0.01 0.00\r\n0.01 0.00 0.01 0.00\r\n0.01 0.01 0.01 0.00\r\n0.01 0.00 0.00 0.00\r\n0.01 0.01 0.01 0.00\r\n0.01 0.01 0.01 0.00\r\n0.00 0.01 0.01 0.00\r\n0.01 0.01 0.01 0.00\r\n0.01 0.02 0.01 0.00\r\n0.01 0.00 0.00 0.00\r\n0.00 0.00 0.00 0.00\r\n0.01 0.01 0.01 0.00\r\n0.01 0.01 0.01 0.00\r\n0.02 0.01 0.01 0.00\r\n0.01 0.01 0.01 0.00\r\n0.01 0.00 0.01 0.00\r\n0.01 0.00 0.01 0.00\r\n0.01 0.01 0.01 0.00\r\n0.01 0.02 0.01 0.00\r\n0.01 0.01 0.01 0.00\r\n0.00 0.01 0.01 0.00\r\n0.01 -0.00 0.00 0.00\r\n0.00 0.00 0.00 0.00\r\n0.00 0.01 0.01 0.00\r\n0.01 0.01 0.01 0.00\r\n0.01 0.00 0.01 0.00\r\n0.01 0.01 0.01 0.00\r\n0.01 0.01 0.01 0.00\r\n0.00 0.00 0.01 0.00\r\n0.01 0.00 0.01 0.00\r\n0.01 0.01 0.01 0.00\r\n0.01 0.01 0.01 0.00\r\n0.00 0.01 0.01 0.00\r\n0.01 0.01 0.01 0.00\r\n0.00 0.00 0.00 0.00\r\n0.01 0.01 0.01 0.00\r\n0.01 0.01 0.01 0.00\r\n0.01 0.01 0.01 0.00\r\n0.01 0.01 0.01 0.00\r\n0.01 0.01 0.00 0.00\r\n0.01 0.01 0.01 0.00\r\n0.01 0.01 0.01 0.00\r\n0.00 0.01 0.01 0.00\r\n0.01 0.00 0.01 0.00\r\n0.00 0.01 0.01 0.00\r\n0.00 0.01 0.01 0.00\r\n-0.00 0.00 0.00 0.00\r\n0.01 0.01 0.00 0.00\r\n0.01 0.00 0.01 0.00\r\n0.01 0.00 0.00 0.00\r\n0.01 0.01 0.01 0.00\r\n0.00 0.01 0.01 0.00\r\n0.00 0.01 0.01 0.00\r\n0.01 0.01 0.01 0.00\r\n0.00 0.01 0.00 0.00\r\n0.01 0.01 0.01 0.00\r\n0.01 0.01 0.01 0.00\r\n0.01 0.01 0.00 0.00\r\n0.01 0.01 0.01 0.00\r\n0.00 0.00 0.00 0.00\r\n0.01 0.01 0.01 0.00\r\n0.01 0.01 0.01 0.00\r\n0.01 0.00 0.01 0.00\r\n0.01 0.01 0.01 0.00\r\n0.01 0.01 0.01 0.00\r\n0.01 0.01 0.01 0.00\r\n0.00 0.01 0.01 0.00\r\n0.01 0.01 0.02 0.00\r\n0.00 0.01 0.00 0.00\r\n-0.00 0.01 0.00 0.00\r\n0.01 0.01 0.01 0.00\r\n0.01 0.01 0.01 0.00\r\n0.00 0.00 0.01 0.00\r\n0.01 0.01 0.01 0.00\r\n0.01 0.00 0.00 0.00\r\n0.00 0.00 -0.00 0.00\r\n0.01 0.01 0.01 0.00\r\n0.01 0.00 0.01 0.00\r\n0.01 0.01 0.01 0.00\r\n0.00 0.01 0.01 0.00\r\n0.01 0.01 0.00 0.00\r\n0.00 0.01 0.00 0.00\r\n0.00 0.01 0.00 0.00\r\n0.01 0.01 0.01 0.00\r\n0.00 0.01 0.01 0.00\r\n0.01 0.01 0.01 0.00\r\n0.00 0.01 0.00 0.00\r\n0.00 0.01 0.01 0.00\r\n0.01 0.01 0.01 0.00\r\n0.00 0.02 0.01 0.00\r\n0.01 0.01 0.01 0.00\r\n0.01 0.01 0.01 0.00\r\n0.01 0.01 0.00 0.00\r\n0.01 0.01 0.00 0.00\r\n-0.00 0.01 0.01 0.00\r\n0.01 -0.00 0.01 0.00\r\n0.01 0.01 0.00 0.00\r\n0.01 0.01 0.01 0.00\r\n0.01 0.01 0.01 0.00\r\n0.01 0.01 0.01 0.00\r\n0.01 0.01 0.01 0.00\r\n0.01 0.00 0.01 0.00\r\n0.00 0.00 0.01 0.00\r\n0.01 0.01 0.01 0.00\r\n0.01 0.01 0.01 0.00\r\n0.00 0.00 0.01 0.00\r\n0.00 0.01 0.01 0.00\r\n0.01 0.01 0.01 0.00\r\n0.01 0.00 0.01 0.00\r\n0.01 0.01 0.01 0.00\r\n0.01 0.01 0.01 0.00\r\n0.01 0.00 0.01 0.00\r\n0.01 0.00 0.01 0.00\r\n0.01 0.01 0.01 0.00\r\n0.01 0.00 0.01 0.00\r\n0.00 0.01 0.01 0.00\r\n0.01 0.01 0.01 0.00\r\n0.01 0.01 0.01 0.00\r\n0.01 0.01 0.01 0.00\r\n0.01 0.00 0.01 0.00\r\n0.01 0.00 0.01 0.00\r\n0.01 0.01 0.01 0.00\r\n0.01 0.01 0.01 0.00\r\n0.01 0.01 0.01 0.00\r\n0.00 0.01 0.01 0.00\r\n0.00 0.01 0.01 0.00\r\n0.01 0.01 0.02 0.00\r\n0.01 -0.00 0.01 0.00\r\n0.00 0.00 0.01 0.00\r\n0.01 0.01 0.00 0.00\r\n0.01 0.00 0.01 0.00\r\n0.01 0.01 0.00 0.00\r\n0.01 0.01 0.01 0.00\r\n0.00 0.00 0.01 0.00\r\n0.01 0.01 0.01 0.00\r\n0.01 0.01 0.01 0.00\r\n0.00 -0.00 0.00 0.00\r\n0.01 0.00 0.01 0.00\r\n0.01 0.01 0.01 0.00\r\n0.01 0.01 0.01 0.00\r\n0.01 0.01 0.01 0.00\r\n0.00 0.01 0.00 0.00\r\n0.01 0.01 0.01 0.00\r\n0.00 0.01 0.00 0.00\r\n0.01 0.01 0.01 0.00\r\n0.00 0.00 0.01 0.00\r\n0.00 0.01 0.00 0.00\r\n0.01 0.00 0.01 0.00\r\n0.01 0.00 0.01 0.00\r\n0.01 0.01 0.00 0.00\r\n0.02 0.00 0.01 0.00\r\n0.01 0.01 0.00 0.00\r\n0.01 0.01 0.01 0.00\r\n0.01 0.01 0.02 0.00\r\n0.00 0.01 0.00 0.00\r\n0.01 0.00 0.01 0.00\r\n0.01 0.01 0.01 0.00\r\n0.01 0.00 0.01 0.00\r\n0.01 0.01 0.01 0.00\r\n0.01 0.01 0.00 0.00\r\n0.01 0.00 0.01 0.00\r\n0.00 0.01 0.01 0.00\r\n0.01 0.01 0.01 0.00\r\n0.01 0.01 0.01 0.00\r\n0.01 0.00 0.01 0.00\r\n0.01 0.01 0.01 0.00\r\n0.00 0.01 0.01 0.00\r\n0.01 0.01 0.01 0.00\r\n0.01 0.01 0.01 0.00\r\n0.01 0.01 0.01 0.00\r\n0.00 0.00 0.01 0.00\r\n0.00 0.00 0.01 0.00\r\n0.01 0.01 0.01 0.00\r\n0.01 0.01 0.00 0.00\r\n0.01 0.01 0.01 0.00\r\n0.01 0.01 0.00 0.00\r\n-0.00 0.01 0.01 0.00\r\n0.01 0.01 0.01 0.00\r\n0.01 0.01 0.00 0.00\r\n0.00 0.01 0.01 0.00\r\n0.00 0.00 0.00 0.00\r\n0.01 0.01 0.01 0.00\r\n0.01 0.01 0.01 0.00\r\n0.01 0.00 0.01 0.00\r\n0.00 0.01 0.01 0.00\r\n0.01 0.01 0.01 0.00\r\n0.00 0.00 0.01 0.00\r\n0.01 0.01 0.01 0.00\r\n0.01 0.00 0.01 0.00\r\n0.01 0.01 0.01 0.00\r\n0.01 0.00 0.00 0.00\r\n0.01 0.01 0.01 0.00\r\n0.01 0.01 0.00 0.00\r\n0.00 0.01 0.01 0.00\r\n0.00 0.01 0.00 0.00\r\n-0.00 0.01 -0.00 0.00\r\n0.01 0.01 0.01 0.00\r\n0.01 0.00 0.01 0.00\r\n0.01 0.01 0.00 0.00\r\n0.01 0.01 0.01 0.00\r\n0.02 0.01 0.01 0.00\r\n0.00 0.00 0.01 0.00\r\n0.01 0.01 0.01 0.00\r\n0.01 0.01 0.01 0.00\r\n0.01 0.01 0.01 0.00\r\n0.01 0.01 0.01 0.00\r\n0.01 0.01 0.01 0.00\r\n0.01 0.00 -0.00 0.00\r\n0.00 0.01 0.01 0.00\r\n0.01 0.00 0.00 0.00\r\n0.00 0.00 0.01 0.00\r\n0.01 0.01 0.01 0.00\r\n0.01 0.01 0.00 0.00\r\n0.00 0.01 0.00 0.00\r\n0.00 0.01 0.01 0.00\r\n0.01 0.01 0.01 0.00\r\n0.00 0.01 0.00 0.00\r\n0.00 -0.00 0.01 0.00\r\n0.01 0.01 0.01 0.00\r\n0.01 0.00 0.00 0.00\r\n0.01 0.01 0.01 0.00\r\n0.01 0.01 0.01 0.00\r\n0.00 0.01 0.01 0.00\r\n0.01 0.01 0.01 0.00\r\n0.00 0.01 0.01 0.00\r\n0.01 0.00 0.01 0.00\r\n0.00 0.01 0.01 0.00\r\n0.01 0.01 0.01 0.00\r\n0.00 0.00 0.00 0.00\r\n0.01 0.01 0.01 0.00\r\n0.01 0.00 0.01 0.00\r\n0.01 0.01 0.00 0.00\r\n0.00 0.00 0.01 0.00\r\n0.01 0.01 0.01 0.00\r\n0.01 0.00 0.01 0.00\r\n0.01 0.01 0.01 0.00\r\n0.01 0.01 0.00 0.00\r\n0.01 0.01 0.01 0.00\r\n-0.00 0.01 -0.00 0.00\r\n0.01 0.01 0.01 0.00\r\n0.01 0.01 0.01 0.00\r\n0.01 0.01 0.01 0.00\r\n0.01 0.00 0.01 0.00\r\n0.01 0.01 0.01 0.00\r\n0.01 0.01 0.01 0.00\r\n0.01 0.01 0.01 0.00\r\n0.01 0.00 -0.00 0.00\r\n-0.00 0.00 0.00 0.00\r\n0.01 0.01 0.01 0.00\r\n0.01 0.01 0.00 0.00\r\n0.01 0.01 0.01 0.00\r\n0.01 0.01 0.01 0.00\r\n0.01 0.01 0.00 0.00\r\n0.01 0.01 0.01 0.00\r\n0.01 0.01 0.01 0.00\r\n0.01 0.01 0.01 0.00\r\n0.01 0.00 0.01 0.00\r\n0.01 0.01 0.01 0.00\r\n0.00 0.01 0.01 0.00\r\n0.01 -0.00 0.01 0.00\r\n0.01 0.01 0.01 0.00\r\n0.01 0.01 0.01 0.00\r\n0.01 0.01 0.00 0.00\r\n0.01 0.01 0.01 0.00\r\n0.02 0.01 0.01 0.00\r\n0.01 0.01 0.01 0.00\r\n0.00 0.01 0.01 0.00\r\n0.01 0.01 0.01 0.00\r\n0.00 0.01 0.00 0.00\r\n0.01 0.00 0.00 0.00\r\n0.01 0.01 0.00 0.00\r\n0.01 -0.00 0.01 0.00\r\n0.00 0.01 0.00 0.00\r\n0.01 0.01 0.01 0.00\r\n0.01 0.00 0.00 0.00\r\n0.00 0.01 0.00 0.00\r\n-0.00 0.01 0.01 0.00\r\n0.00 0.00 0.00 0.00\r\n0.01 0.01 0.01 0.00\r\n0.01 0.01 0.01 0.00\r\n0.01 0.00 0.01 0.00\r\n0.00 0.00 0.00 0.00\r\n0.01 0.01 0.01 0.00\r\n0.01 0.01 0.01 0.00\r\n0.01 0.01 0.01 0.00\r\n0.01 0.01 0.01 0.00\r\n0.00 0.00 0.00 0.00\r\n0.01 0.01 0.01 0.00\r\n0.01 0.01 0.01 0.00\r\n0.01 0.00 0.01 0.00\r\n-0.00 0.00 0.00 0.00\r\n0.01 0.01 0.01 0.00\r\n0.01 0.00 0.01 0.00\r\n0.01 0.01 0.01 0.00\r\n0.01 0.00 0.01 0.00\r\n0.01 0.00 0.00 0.00\r\n0.01 0.01 0.00 0.00\r\n0.01 0.01 0.01 0.00\r\n0.01 0.01 0.01 0.00\r\n0.01 0.01 0.00 0.00\r\n0.01 0.01 0.01 0.00\r\n0.01 0.01 0.01 0.00\r\n0.00 0.01 0.01 0.00\r\n0.01 0.01 0.01 0.00\r\n0.00 0.01 0.00 0.00\r\n0.01 0.00 0.00 0.00\r\n0.01 0.01 0.00 0.00\r\n0.01 0.01 0.01 0.00\r\n0.01 0.00 0.01 0.00\r\n0.01 0.00 0.01 0.00\r\n0.01 0.01 0.01 0.00\r\n0.01 0.01 0.00 0.00\r\n0.01 0.01 0.01 0.00\r\n0.01 0.00 0.01 0.00\r\n0.00 0.01 0.00 0.00\r\n0.01 0.01 0.01 0.00\r\n0.01 0.01 0.00 0.00\r\n0.01 -0.00 0.00 0.00\r\n0.01 0.01 0.01 0.00\r\n0.01 0.01 0.00 0.00\r\n0.00 0.01 0.01 0.00\r\n0.00 0.00 0.01 0.00\r\n0.01 0.01 0.01 0.00\r\n0.01 0.01 0.01 0.00\r\n0.01 0.01 0.01 0.00\r\n0.01 0.01 0.01 0.00\r\n0.01 0.00 0.01 0.00\r\n0.00 0.01 0.00 0.00\r\n0.01 0.01 0.01 0.00\r\n0.01 0.01 0.00 0.00\r\n0.00 0.01 0.00 0.00\r\n0.01 0.01 0.01 0.00\r\n0.01 0.00 0.01 0.00\r\n0.00 0.01 0.00 0.00\r\n0.01 0.01 0.01 0.00\r\n0.01 0.00 0.01 0.00\r\n0.01 0.01 0.01 0.00\r\n0.01 0.01 0.01 0.00\r\n0.01 0.01 0.01 0.00\r\n0.00 0.00 0.00 0.00\r\n0.00 0.01 0.01 0.00\r\n0.01 0.01 0.01 0.00\r\n0.00 0.01 0.01 0.00\r\n0.00 0.01 0.01 0.00\r\n0.01 0.01 0.00 0.00\r\n0.00 0.01 0.01 0.00\r\n0.01 0.01 0.01 0.00\r\n0.01 0.00 0.01 0.00\r\n0.01 0.00 0.01 0.00\r\n0.01 0.01 0.01 0.00\r\n0.01 0.01 0.01 0.00\r\n0.01 0.01 0.01 0.00\r\n0.00 0.01 0.00 0.00\r\n0.01 0.01 0.00 0.00\r\n0.00 0.01 0.00 0.00\r\n0.01 0.01 0.02 0.00\r\n0.01 0.01 0.00 0.00\r\n0.00 0.01 0.00 0.00\r\n0.00 0.01 0.00 0.00\r\n0.01 0.00 0.01 0.00\r\n0.01 0.01 0.01 0.00\r\n0.01 0.01 0.00 0.00\r\n0.00 0.00 0.01 0.00\r\n0.00 -0.00 -0.00 0.00\r\n0.00 0.01 0.01 0.00\r\n0.01 0.00 -0.00 0.00\r\n0.01 0.01 0.01 0.00\r\n0.01 0.00 0.00 0.00\r\n0.01 0.01 0.01 0.00\r\n0.01 0.00 0.01 0.00\r\n0.01 0.00 0.01 0.00\r\n0.01 0.01 0.00 0.00\r\n0.01 0.01 0.02 0.00\r\n0.01 0.01 0.01 0.00\r\n0.00 0.01 0.01 0.00\r\n0.01 0.01 0.01 0.00\r\n0.00 0.00 0.00 0.00\r\n0.00 0.01 0.01 0.00\r\n0.01 0.01 0.01 0.00\r\n0.00 0.00 0.01 0.00\r\n0.00 0.01 0.00 0.00\r\n0.01 0.01 0.01 0.00\r\n0.01 0.01 0.01 0.00\r\n0.00 0.01 0.01 0.00\r\n0.01 0.00 0.00 0.00\r\n0.01 0.01 0.01 0.00\r\n0.01 0.01 0.01 0.00\r\n0.01 0.00 0.01 0.00\r\n0.00 0.00 0.00 0.00\r\n0.01 0.01 0.01 0.00\r\n0.00 0.00 0.00 0.00\r\n0.01 0.01 0.00 0.00\r\n0.01 0.01 0.01 0.00\r\n0.01 0.00 0.01 0.00\r\n0.00 0.00 0.01 0.00\r\n0.01 0.00 0.01 0.00\r\n0.00 0.01 0.01 0.00\r\n0.00 0.00 0.00 0.00\r\n0.01 0.01 0.01 0.00\r\n0.01 0.00 0.01 0.00\r\n0.01 0.01 0.00 0.00\r\n0.00 0.01 0.00 0.00\r\n0.01 0.01 0.01 0.00\r\n0.01 0.00 0.01 0.00\r\n0.01 0.01 0.01 0.00\r\n0.01 0.00 0.01 0.00\r\n0.00 0.00 0.01 0.00\r\n0.01 0.00 0.00 0.00\r\n0.01 0.01 0.01 0.00\r\n0.01 0.01 0.01 0.00\r\n0.01 0.01 0.01 0.00\r\n0.01 0.01 0.01 0.00\r\n0.01 0.00 0.00 0.00\r\n0.00 0.01 0.01 0.00\r\n0.00 0.01 0.01 0.00\r\n0.01 0.00 -0.00 0.00\r\n0.01 0.00 0.00 0.00\r\n0.01 0.01 0.01 0.00\r\n0.01 0.01 0.01 0.00\r\n0.00 0.01 0.00 0.00\r\n0.00 0.01 0.01 0.00\r\n0.01 0.00 0.01 0.00\r\n0.00 0.01 0.00 0.00\r\n0.01 0.01 0.01 0.00\r\n0.01 0.01 0.01 0.00\r\n0.00 0.01 0.01 0.00\r\n0.00 0.00 0.01 0.00\r\n0.01 0.01 0.01 0.00\r\n0.01 0.01 0.00 0.00\r\n0.01 0.01 0.01 0.00\r\n0.00 -0.00 0.00 0.00\r\n0.02 0.00 0.01 0.00\r\n0.01 0.01 0.01 0.00\r\n0.01 0.01 0.01 0.00\r\n0.01 0.01 0.00 0.00\r\n0.01 0.01 0.01 0.00\r\n0.01 0.01 0.01 0.00\r\n0.00 0.01 0.01 0.00\r\n0.01 0.01 0.01 0.00\r\n0.01 0.01 0.01 0.00\r\n0.00 0.01 0.01 0.00\r\n0.00 0.01 0.01 0.00\r\n0.01 0.01 0.01 0.00\r\n0.01 0.01 0.00 0.00\r\n0.00 0.01 0.01 0.00\r\n0.01 0.01 0.01 0.00\r\n0.01 0.01 0.01 0.00\r\n0.00 0.01 0.01 0.00\r\n0.01 0.01 0.01 0.00\r\n0.01 0.01 0.01 0.00\r\n0.01 0.00 0.01 0.00\r\n0.01 0.01 0.01 0.00\r\n0.01 0.01 0.01 0.00\r\n0.01 0.01 0.01 0.00\r\n0.01 0.01 0.01 0.00\r\n0.00 0.01 0.01 0.00\r\n0.01 0.01 0.01 0.00\r\n0.01 0.01 0.01 0.00\r\n0.01 0.00 0.01 0.00\r\n0.00 0.00 0.00 0.00\r\n0.00 0.01 0.01 0.00\r\n0.01 0.00 0.01 0.00\r\n0.01 0.00 0.01 0.00\r\n0.01 0.01 0.01 0.00\r\n0.01 0.00 0.01 0.00\r\n0.01 0.01 0.01 0.00\r\n0.01 0.01 0.01 0.00\r\n0.01 0.01 0.01 0.00\r\n0.02 0.00 0.01 0.00\r\n0.01 0.01 0.01 0.00\r\n0.01 0.01 0.01 0.00\r\n0.01 0.00 0.00 0.00\r\n0.01 0.01 0.01 0.00\r\n0.01 0.01 0.01 0.00\r\n0.01 0.01 0.01 0.00\r\n0.01 0.01 0.01 0.00\r\n0.01 0.00 0.01 0.00\r\n0.01 0.00 0.00 0.00\r\n0.00 0.01 0.01 0.00\r\n0.00 0.01 0.01 0.00\r\n0.01 0.01 0.01 0.00\r\n0.01 0.01 0.01 0.00\r\n0.01 0.01 0.01 0.00\r\n0.00 0.01 0.01 0.00\r\n0.01 0.01 0.01 0.00\r\n0.01 0.01 0.01 0.00\r\n0.00 0.01 0.01 0.00\r\n0.01 0.01 0.01 0.00\r\n0.01 0.01 0.01 0.00\r\n0.01 0.00 0.01 0.00\r\n0.01 0.02 0.01 0.00\r\n0.00 0.00 0.01 0.00\r\n0.01 0.01 0.01 0.00\r\n0.01 0.00 0.00 0.00\r\n0.01 0.01 0.01 0.00\r\n0.00 0.00 0.01 0.00\r\n0.01 0.01 0.01 0.00\r\n0.01 0.01 0.00 0.00\r\n0.01 0.00 0.01 0.00\r\n0.01 0.00 0.00 0.00\r\n0.01 0.01 0.00 0.00\r\n0.01 0.00 0.01 0.00\r\n0.00 0.01 -0.00 0.00\r\n0.01 0.01 0.01 0.00\r\n0.01 0.01 0.01 0.00\r\n0.01 0.00 0.01 0.00\r\n0.01 0.01 0.01 0.00\r\n0.01 0.01 0.01 0.00\r\n0.01 0.00 0.01 0.00\r\n0.00 0.01 0.01 0.00\r\n0.01 0.00 0.01 0.00\r\n0.00 0.00 0.00 0.00\r\n0.00 0.01 0.01 0.00\r\n0.01 0.01 0.00 0.00\r\n0.01 0.01 0.01 0.00\r\n0.01 0.02 0.01 0.00\r\n0.00 0.01 -0.00 0.00\r\n0.01 0.01 0.01 0.00\r\n0.01 0.01 0.00 0.00\r\n0.01 0.01 0.01 0.00\r\n0.01 0.00 0.01 0.00\r\n0.01 0.01 0.01 0.00\r\n0.01 0.01 0.01 0.00\r\n0.01 0.00 0.01 0.00\r\n0.01 0.01 0.01 0.00\r\n0.00 0.01 0.00 0.00\r\n0.01 0.01 0.01 0.00\r\n0.00 0.00 0.00 0.00\r\n0.01 0.00 0.01 0.00\r\n0.01 -0.00 0.00 0.00\r\n0.01 0.01 0.01 0.00\r\n0.01 0.01 0.01 0.00\r\n0.01 0.00 0.01 0.00\r\n0.00 0.00 0.00 0.00\r\n0.00 0.01 0.00 0.00\r\n0.00 0.01 0.00 0.00\r\n0.01 -0.00 -0.00 0.00\r\n0.01 0.01 0.01 0.00\r\n0.01 0.01 0.01 0.00\r\n0.00 0.01 0.00 0.00\r\n0.01 0.01 0.01 0.00\r\n0.00 0.01 0.01 0.00\r\n0.01 0.01 0.00 0.00\r\n0.01 0.01 0.01 0.00\r\n0.01 0.01 0.01 0.00\r\n0.00 0.00 0.01 0.00\r\n0.01 0.01 0.01 0.00\r\n0.01 0.01 0.01 0.00\r\n0.01 0.01 0.01 0.00\r\n0.00 0.01 0.00 0.00\r\n0.01 0.00 0.01 0.00\r\n0.00 0.01 0.00 0.00\r\n0.01 0.01 0.01 0.00\r\n0.01 0.00 0.01 0.00\r\n0.01 0.01 0.00 0.00\r\n0.01 0.01 0.01 0.00\r\n0.01 0.00 0.00 0.00\r\n0.01 0.00 0.00 0.00\r\n0.01 0.01 0.01 0.00\r\n0.00 0.01 0.01 0.00\r\n0.00 0.01 0.00 0.00\r\n0.00 0.01 0.01 0.00\r\n0.00 0.01 0.01 0.00\r\n0.00 0.00 0.01 0.00\r\n0.00 0.01 0.00 0.00\r\n0.01 0.01 0.01 0.00\r\n0.01 0.01 0.00 0.00\r\n0.00 0.00 0.00 0.00\r\n0.02 0.00 0.01 0.00\r\n0.01 0.01 0.01 0.00\r\n0.00 0.00 0.00 0.00\r\n0.00 0.01 0.01 0.00\r\n0.01 0.00 0.00 0.00\r\n0.01 0.01 0.01 0.00\r\n0.01 0.01 0.00 0.00\r\n0.00 0.01 0.00 0.00\r\n0.01 0.00 0.00 0.00\r\n0.01 0.01 0.01 0.00\r\n0.01 0.01 0.01 0.00\r\n0.00 0.01 0.01 0.00\r\n0.00 0.01 -0.00 0.00\r\n0.01 0.01 0.01 0.00\r\n0.00 0.01 0.01 0.00\r\n0.01 0.01 0.01 0.00\r\n0.01 0.00 0.01 0.00\r\n0.01 0.00 -0.00 0.00\r\n0.01 0.01 0.01 0.00\r\n0.01 0.01 0.01 0.00\r\n0.01 0.01 0.01 0.00\r\n0.01 0.01 0.00 0.00\r\n0.02 0.01 0.01 0.00\r\n0.00 0.00 0.01 0.00\r\n0.01 0.01 0.01 0.00\r\n0.01 0.00 0.00 0.00\r\n0.00 0.01 0.01 0.00\r\n0.01 0.01 0.00 0.00\r\n0.01 0.01 0.01 0.00\r\n0.01 0.00 0.01 0.00\r\n-0.00 0.01 0.01 0.00\r\n0.01 0.00 0.00 0.00\r\n0.01 0.01 0.01 0.00\r\n0.00 0.01 0.01 0.00\r\n0.01 0.01 0.01 0.00\r\n0.00 0.00 0.01 0.00\r\n0.00 0.01 0.01 0.00\r\n0.01 0.01 0.01 0.00\r\n0.01 0.01 0.01 0.00\r\n0.01 0.01 0.00 0.00\r\n0.01 0.00 0.01 0.00\r\n0.01 0.01 0.00 0.00\r\n0.01 0.01 0.01 0.00\r\n0.01 0.01 0.01 0.00\r\n0.01 0.01 0.00 0.00\r\n0.01 0.01 0.01 0.00\r\n0.00 0.01 0.00 0.00\r\n0.01 0.01 0.01 0.00\r\n0.00 0.01 0.00 0.00\r\n0.01 0.01 0.00 0.00\r\n0.00 0.01 0.01 0.00\r\n0.01 0.01 0.01 0.00\r\n0.01 0.01 0.01 0.00\r\n0.01 0.00 0.00 0.00\r\n0.01 0.01 0.01 0.00\r\n0.00 0.01 0.01 0.00\r\n0.01 0.01 0.01 0.00\r\n0.00 0.01 0.00 0.00\r\n0.00 -0.00 0.00 0.00\r\n0.01 0.01 0.01 0.00\r\n0.01 0.00 0.01 0.00\r\n0.01 0.00 0.01 0.00\r\n0.00 0.01 0.01 0.00\r\n0.00 0.01 0.00 0.00\r\n0.00 0.01 0.01 0.00\r\n0.01 0.01 0.01 0.00\r\n0.01 0.00 0.00 0.00\r\n0.01 0.01 0.01 0.00\r\n0.01 0.01 0.01 0.00\r\n0.01 0.00 0.01 0.00\r\n0.00 0.01 0.01 0.00\r\n0.01 0.01 0.01 0.00\r\n0.00 0.00 0.01 0.00\r\n0.01 0.00 -0.00 0.00\r\n0.01 0.01 0.01 0.00\r\n0.01 0.01 0.01 0.00\r\n0.01 0.01 0.01 0.00\r\n0.00 0.00 0.01 0.00\r\n-0.00 0.00 0.00 0.00\r\n0.01 0.01 0.01 0.00\r\n0.01 0.01 0.02 0.00\r\n0.00 0.01 0.01 0.00\r\n0.00 0.01 0.00 0.00\r\n0.01 0.01 0.00 0.00\r\n0.01 0.01 0.00 0.00\r\n0.01 0.01 0.01 0.00\r\n0.01 0.01 0.01 0.00\r\n0.01 0.00 0.00 0.00\r\n0.00 0.01 -0.00 0.00\r\n0.01 0.01 0.01 0.00\r\n0.01 0.01 0.01 0.00\r\n0.00 0.01 0.00 0.00\r\n0.01 0.01 0.01 0.00\r\n-0.00 0.01 0.01 0.00\r\n0.00 -0.00 0.00 0.00\r\n0.01 0.01 0.01 0.00\r\n0.01 0.01 0.01 0.00\r\n0.01 0.00 0.01 0.00\r\n0.00 0.01 0.01 0.00\r\n0.00 0.01 0.00 0.00\r\n0.01 0.00 0.00 0.00\r\n0.01 0.01 0.01 0.00\r\n0.01 0.00 0.01 0.00\r\n0.01 0.01 0.01 0.00\r\n0.00 0.01 0.01 0.00\r\n0.01 0.01 0.01 0.00\r\n0.00 0.01 0.00 0.00\r\n0.02 0.01 0.01 0.00\r\n0.01 0.01 0.01 0.00\r\n0.01 0.00 0.00 0.00\r\n0.00 0.00 0.01 0.00\r\n0.01 0.01 0.00 0.00\r\n0.01 0.01 0.01 0.00\r\n0.00 0.01 0.00 0.00\r\n0.01 0.01 0.01 0.00\r\n0.00 0.00 0.01 0.00\r\n0.01 0.01 0.01 0.00\r\n0.00 0.00 0.01 0.00\r\n0.01 0.01 0.01 0.00\r\n0.01 0.01 0.01 0.00\r\n0.01 0.01 0.01 0.00\r\n0.00 0.01 0.00 0.00\r\n0.00 0.00 0.00 0.00\r\n0.01 0.01 0.01 0.00\r\n0.01 0.01 0.01 0.00\r\n0.01 0.01 0.01 0.00\r\n0.00 0.01 0.00 0.00\r\n0.01 -0.00 0.01 0.00\r\n0.00 0.01 0.01 0.00\r\n0.01 0.00 0.01 0.00\r\n0.01 0.01 0.01 0.00\r\n0.01 0.01 0.01 0.00\r\n0.01 0.01 0.00 0.00\r\n0.01 0.01 0.01 0.00\r\n0.01 0.01 0.01 0.00\r\n0.00 0.01 0.00 0.00\r\n0.01 0.00 0.01 0.00\r\n0.00 0.01 0.00 0.00\r\n0.01 0.01 0.01 0.00\r\n0.01 0.01 0.00 0.00\r\n0.00 0.01 0.01 0.00\r\n0.01 0.01 0.01 0.00\r\n0.01 0.01 0.01 0.00\r\n0.01 0.01 0.01 0.00\r\n0.01 0.01 0.01 0.00\r\n0.01 0.01 0.01 0.00\r\n0.01 0.00 0.01 0.00\r\n0.01 0.01 0.01 0.00\r\n0.01 0.01 0.01 0.00\r\n0.01 0.01 0.01 0.00\r\n0.00 0.01 0.01 0.00\r\n0.00 0.01 0.01 0.00\r\n0.01 0.00 0.01 0.00\r\n0.01 0.01 0.01 0.00\r\n0.01 0.01 0.00 0.00\r\n0.01 0.01 0.01 0.00\r\n0.01 0.01 0.01 0.00\r\n0.00 0.01 0.01 0.00\r\n0.01 0.01 0.01 0.00\r\n0.00 0.01 0.01 0.00\r\n0.00 0.01 0.01 0.00\r\n0.01 0.00 0.01 0.00\r\n0.01 0.01 0.01 0.00\r\n0.01 0.01 0.01 0.00\r\n0.00 0.00 0.01 0.00\r\n0.00 0.01 0.01 0.00\r\n0.01 0.01 0.01 0.00\r\n0.01 0.01 0.01 0.00\r\n0.00 0.01 0.01 0.00\r\n0.01 0.00 0.00 0.00\r\n0.01 0.01 0.01 0.00\r\n0.00 0.01 0.00 0.00\r\n0.01 0.01 0.01 0.00\r\n0.01 0.00 0.01 0.00\r\n0.01 0.00 0.00 0.00\r\n0.01 0.01 0.01 0.00\r\n0.01 0.00 0.01 0.00\r\n0.01 0.00 0.00 0.00\r\n0.01 0.01 0.01 0.00\r\n0.01 0.00 0.00 0.00\r\n0.00 0.01 0.00 0.00\r\n0.01 0.01 0.01 0.00\r\n0.01 0.01 0.01 0.00\r\n0.01 0.00 0.00 0.00\r\n0.02 0.01 0.01 0.00\r\n0.01 0.02 0.01 0.00\r\n0.01 0.01 0.01 0.00\r\n0.01 0.01 0.01 0.00\r\n0.01 0.01 0.00 0.00\r\n-0.00 0.01 0.00 0.00\r\n0.01 0.01 0.01 0.00\r\n0.01 0.01 0.01 0.00\r\n0.00 0.00 0.00 0.00\r\n-0.00 0.01 0.00 0.00\r\n0.01 0.01 0.01 0.00\r\n0.01 0.01 0.01 0.00\r\n0.01 0.01 0.01 0.00\r\n0.01 0.01 0.00 0.00\r\n0.01 0.01 0.01 0.00\r\n0.01 0.01 0.00 0.00\r\n0.01 0.01 0.01 0.00\r\n0.00 0.01 0.00 0.00\r\n0.01 0.00 0.01 0.00\r\n0.01 0.01 0.01 0.00\r\n0.01 0.01 0.01 0.00\r\n-0.00 0.01 0.01 0.00\r\n0.01 0.01 0.01 0.00\r\n0.00 0.01 0.01 0.00\r\n0.00 0.01 0.01 0.00\r\n0.01 0.01 0.01 0.00\r\n0.01 0.01 0.01 0.00\r\n0.01 0.00 -0.00 0.00\r\n0.01 0.01 0.01 0.00\r\n0.01 0.01 0.01 0.00\r\n0.01 0.01 0.00 0.00\r\n0.01 0.02 0.02 0.00\r\n0.01 -0.00 0.01 0.00\r\n0.01 0.01 0.01 0.00\r\n0.00 0.01 0.00 0.00\r\n0.01 0.01 0.01 0.00\r\n0.01 0.00 0.00 0.00\r\n0.01 0.01 0.01 0.00\r\n0.01 0.01 0.01 0.00\r\n0.00 0.01 0.00 0.00\r\n0.01 0.01 0.01 0.00\r\n0.01 0.01 0.01 0.00\r\n0.00 0.01 0.01 0.00\r\n0.01 0.01 0.01 0.00\r\n0.01 0.01 0.01 0.00\r\n0.01 0.01 0.01 0.00\r\n0.00 0.01 0.00 0.00\r\n0.01 0.01 0.01 0.00\r\n0.01 0.01 0.01 0.00\r\n-0.00 0.01 0.01 0.00\r\n0.01 0.00 0.00 0.00\r\n0.01 0.00 0.01 0.00\r\n0.00 0.00 0.00 0.00\r\n0.01 0.00 0.00 0.00\r\n0.00 0.01 0.01 0.00\r\n0.01 0.01 0.01 0.00\r\n0.02 0.01 0.01 0.00\r\n0.00 0.00 0.01 0.00\r\n0.01 0.01 0.01 0.00\r\n0.01 0.00 0.01 0.00\r\n0.01 0.00 0.00 0.00\r\n0.01 0.01 0.00 0.00\r\n-0.00 0.01 0.01 0.00\r\n0.01 0.00 0.00 0.00\r\n0.00 0.00 0.00 0.00\r\n0.01 0.01 0.01 0.00\r\n0.00 -0.00 0.01 0.00\r\n0.00 0.01 0.01 0.00\r\n0.01 0.01 0.01 0.00\r\n0.01 0.01 0.01 0.00\r\n0.01 0.00 0.01 0.00\r\n0.01 0.00 0.01 0.00\r\n0.01 0.00 0.00 0.00\r\n0.01 0.01 0.01 0.00\r\n0.01 0.00 0.01 0.00\r\n0.01 0.01 0.01 0.00\r\n0.01 0.01 0.01 0.00\r\n0.01 0.01 0.01 0.00\r\n0.00 0.01 0.00 0.00\r\n0.01 0.01 0.01 0.00\r\n0.01 0.01 0.01 0.00\r\n0.01 0.01 0.01 0.00\r\n0.01 0.00 0.01 0.00\r\n0.01 0.01 0.01 0.00\r\n0.01 0.01 0.01 0.00\r\n0.00 0.01 0.00 0.00\r\n0.01 0.00 0.00 0.00\r\n0.01 0.01 0.01 0.00\r\n0.01 0.00 0.00 0.00\r\n0.01 0.00 0.00 0.00\r\n0.01 0.01 0.01 0.00\r\n0.01 0.01 0.01 0.00\r\n0.01 0.01 0.01 0.00\r\n0.01 0.01 0.01 0.00\r\n-0.00 0.00 0.00 0.00\r\n0.01 0.00 0.00 0.00\r\n0.01 0.01 0.01 0.00\r\n0.01 0.01 0.00 0.00\r\n0.00 0.01 0.01 0.00\r\n0.00 0.01 0.01 0.00\r\n0.00 0.00 0.00 0.00\r\n0.01 0.01 0.00 0.00\r\n0.01 0.01 0.01 0.00\r\n0.01 0.01 0.01 0.00\r\n0.00 0.01 0.01 0.00\r\n0.01 0.01 0.01 0.00\r\n0.01 0.01 0.01 0.00\r\n0.01 0.01 0.01 0.00\r\n0.01 0.01 0.01 0.00\r\n0.01 0.01 0.01 0.00\r\n0.00 0.00 0.01 0.00\r\n0.01 0.00 0.01 0.00\r\n0.01 0.01 0.01 0.00\r\n0.01 0.01 0.01 0.00\r\n0.01 0.01 0.01 0.00\r\n0.01 0.01 0.01 0.00\r\n-0.00 0.01 0.00 0.00\r\n0.00 0.01 0.01 0.00\r\n0.01 0.00 0.01 0.00\r\n0.01 0.01 0.01 0.00\r\n0.00 0.00 0.01 0.00\r\n0.01 0.01 0.01 0.00\r\n0.00 0.00 0.00 0.00\r\n0.01 0.01 0.00 0.00\r\n0.01 0.01 0.00 0.00\r\n0.00 0.00 0.01 0.00\r\n0.01 0.01 0.01 0.00\r\n0.01 0.01 0.01 0.00\r\n0.01 0.01 0.01 0.00\r\n0.01 0.01 0.01 0.00\r\n0.01 0.00 0.01 0.00\r\n0.01 0.01 0.01 0.00\r\n0.00 0.01 0.01 0.00\r\n0.01 0.01 0.01 0.00\r\n0.01 0.01 0.01 0.00\r\n0.00 0.01 0.01 0.00\r\n0.01 0.01 0.01 0.00\r\n0.00 0.01 0.00 0.00\r\n0.01 0.00 0.01 0.00\r\n0.01 0.01 0.01 0.00\r\n0.00 0.00 0.00 0.00\r\n0.00 0.01 0.00 0.00\r\n0.01 0.01 0.01 0.00\r\n0.00 0.00 0.00 0.00\r\n0.01 0.01 0.00 0.00\r\n0.01 0.00 0.01 0.00\r\n0.00 0.01 0.01 0.00\r\n0.01 0.00 0.00 0.00\r\n0.01 0.01 0.01 0.00\r\n0.00 0.01 0.01 0.00\r\n0.01 0.01 0.01 0.00\r\n0.01 0.00 0.01 0.00\r\n0.01 0.00 0.00 0.00\r\n0.00 0.01 0.00 0.00\r\n0.01 0.01 0.01 0.00\r\n0.01 0.01 0.00 0.00\r\n0.00 0.01 0.01 0.00\r\n0.02 0.00 0.01 0.00\r\n0.01 0.01 0.01 0.00\r\n0.01 0.01 0.00 0.00\r\n0.01 0.01 0.01 0.00\r\n0.01 0.00 0.01 0.00\r\n0.00 0.01 0.01 0.00\r\n0.01 0.01 0.01 0.00\r\n0.01 0.00 0.00 0.00\r\n0.01 0.01 0.00 0.00\r\n0.01 0.01 0.01 0.00\r\n0.01 0.01 0.01 0.00\r\n-0.00 0.00 0.00 0.00\r\n0.01 0.00 0.00 0.00\r\n0.01 0.01 0.01 0.00\r\n0.01 0.00 -0.00 0.00\r\n0.01 0.01 0.01 0.00\r\n0.01 0.01 0.00 0.00\r\n0.00 0.01 -0.00 0.00\r\n0.01 0.01 0.01 0.00\r\n0.01 0.00 0.01 0.00\r\n0.01 0.01 0.01 0.00\r\n0.00 0.01 0.00 0.00\r\n0.01 0.00 0.01 0.00\r\n0.00 0.00 0.00 0.00\r\n0.00 0.01 0.01 0.00\r\n0.01 0.01 0.00 0.00\r\n0.01 0.01 0.01 0.00\r\n0.01 0.00 0.01 0.00\r\n0.01 0.01 0.01 0.00\r\n0.01 0.01 0.01 0.00\r\n0.01 0.01 0.01 0.00\r\n0.00 0.01 0.01 0.00\r\n0.01 0.01 0.00 0.00\r\n0.01 0.00 0.01 0.00\r\n0.00 0.01 0.01 0.00\r\n0.00 0.00 0.00 0.00\r\n0.00 0.00 0.00 0.00\r\n0.00 0.01 0.00 0.00\r\n0.00 0.01 0.00 0.00\r\n0.01 0.01 0.01 0.00\r\n0.01 0.01 0.01 0.00\r\n0.01 0.01 0.01 0.00\r\n0.00 0.00 -0.00 0.00\r\n0.01 0.01 0.01 0.00\r\n0.01 0.01 0.01 0.00\r\n0.01 0.01 0.01 0.00\r\n0.01 0.01 0.00 0.00\r\n0.00 0.01 0.01 0.00\r\n0.01 0.00 0.01 0.00\r\n0.00 0.01 0.01 0.00\r\n0.01 0.00 0.00 0.00\r\n0.01 0.01 0.01 0.00\r\n0.00 0.01 0.01 0.00\r\n0.01 0.01 0.01 0.00\r\n0.00 0.01 0.01 0.00\r\n0.00 0.01 0.01 0.00\r\n0.01 0.01 0.00 0.00\r\n0.00 0.01 0.00 0.00\r\n0.01 0.00 0.00 0.00\r\n0.01 0.01 0.00 0.00\r\n0.01 -0.00 0.00 0.00\r\n0.01 0.01 0.01 0.00\r\n0.01 0.01 0.01 0.00\r\n0.00 0.01 0.00 0.00\r\n0.00 0.00 0.00 0.00\r\n0.01 0.00 0.00 0.00\r\n0.00 0.01 0.00 0.00\r\n0.00 0.00 0.01 0.00\r\n0.01 0.01 0.01 0.00\r\n0.01 0.00 0.00 0.00\r\n0.01 0.01 0.01 0.00\r\n0.01 0.01 0.01 0.00\r\n0.01 0.00 0.00 0.00\r\n0.00 0.01 0.01 0.00\r\n0.01 0.01 0.01 0.00\r\n0.01 0.00 0.00 0.00\r\n0.00 0.01 0.01 0.00\r\n0.01 0.01 0.00 0.00\r\n0.01 0.00 0.01 0.00\r\n0.00 0.01 0.00 0.00\r\n0.01 0.01 0.01 0.00\r\n0.01 0.00 0.01 0.00\r\n0.01 0.01 0.01 0.00\r\n0.01 0.01 0.01 0.00\r\n0.01 0.01 0.01 0.00\r\n0.01 0.00 0.01 0.00\r\n0.00 0.01 0.01 0.00\r\n0.01 0.01 0.00 0.00\r\n0.00 0.01 0.01 0.00\r\n0.02 0.01 0.01 0.00\r\n0.01 0.01 0.00 0.00\r\n0.01 0.01 0.00 0.00\r\n0.01 0.01 0.01 0.00\r\n0.01 0.01 0.00 0.00\r\n0.01 0.01 0.01 0.00\r\n0.00 0.00 0.00 0.00\r\n0.00 0.01 0.01 0.00\r\n0.01 0.01 0.00 0.00\r\n0.01 0.01 0.01 0.00\r\n0.01 0.01 0.01 0.00\r\n0.00 0.01 0.01 0.00\r\n0.01 0.00 0.01 0.00\r\n0.01 0.01 0.01 0.00\r\n0.01 0.00 0.00 0.00\r\n0.01 0.01 0.00 0.00\r\n0.01 0.01 0.01 0.00\r\n0.01 0.01 0.01 0.00\r\n0.01 0.00 0.01 0.00\r\n0.01 0.01 0.01 0.00\r\n0.00 0.01 0.00 0.00\r\n0.00 0.01 0.01 0.00\r\n0.01 0.00 0.01 0.00\r\n0.01 0.00 0.01 0.00\r\n0.00 0.01 0.00 0.00\r\n0.00 0.01 0.01 0.00\r\n0.01 0.01 0.01 0.00\r\n0.01 0.01 0.01 0.00\r\n0.00 0.01 0.00 0.00\r\n0.00 0.01 0.01 0.00\r\n0.01 0.00 0.00 0.00\r\n0.01 0.01 0.01 0.00\r\n0.00 0.00 0.00 0.00\r\n0.01 0.01 0.01 0.00\r\n0.01 0.02 0.01 0.00\r\n0.00 0.00 0.00 0.00\r\n0.00 0.00 0.00 0.00\r\n0.00 0.00 0.00 0.00\r\n0.00 0.00 0.00 0.00\r\n0.01 0.00 0.00 0.00\r\n0.01 0.01 0.01 0.00\r\n0.01 0.00 0.01 0.00\r\n0.01 0.00 0.00 0.00\r\n0.01 0.01 0.02 0.00\r\n0.01 0.00 0.00 0.00\r\n0.00 0.01 0.01 0.00\r\n0.01 0.01 0.00 0.00\r\n0.00 0.01 0.00 0.00\r\n0.01 0.01 0.01 0.00\r\n0.01 0.01 0.01 0.00\r\n0.01 0.01 0.01 0.00\r\n0.01 0.01 0.01 0.00\r\n0.00 0.01 0.01 0.00\r\n0.02 0.01 0.01 0.00\r\n0.01 0.01 0.01 0.00\r\n0.01 0.01 0.01 0.00\r\n0.01 0.01 0.01 0.00\r\n0.00 0.01 0.00 0.00\r\n0.01 0.01 0.01 0.00\r\n0.01 0.00 0.01 0.00\r\n0.00 0.00 -0.00 0.00\r\n0.01 0.01 0.01 0.00\r\n0.00 0.00 0.00 0.00\r\n0.01 0.00 0.00 0.00\r\n0.01 0.00 0.01 0.00\r\n0.01 0.01 0.01 0.00\r\n0.01 0.00 0.00 0.00\r\n0.01 0.01 0.01 0.00\r\n0.01 0.01 0.01 0.00\r\n0.00 0.01 0.01 0.00\r\n0.01 0.01 0.01 0.00\r\n0.01 0.01 0.01 0.00\r\n0.01 0.01 0.00 0.00\r\n0.01 0.01 0.01 0.00\r\n0.01 0.01 0.01 0.00\r\n0.01 0.01 0.02 0.00\r\n0.00 0.00 0.00 0.00\r\n0.01 0.00 0.01 0.00\r\n0.01 0.01 0.01 0.00\r\n0.01 0.00 0.01 0.00\r\n0.01 0.01 0.01 0.00\r\n0.00 0.01 0.00 0.00\r\n0.01 0.01 0.01 0.00\r\n0.00 0.01 0.01 0.00\r\n0.01 0.01 0.01 0.00\r\n0.00 0.01 0.01 0.00\r\n0.00 0.01 0.01 0.00\r\n0.01 0.00 0.00 0.00\r\n0.01 0.00 0.01 0.00\r\n0.01 0.01 0.00 0.00\r\n0.01 0.01 0.00 0.00\r\n0.01 0.00 0.01 0.00\r\n0.01 0.01 0.01 0.00\r\n0.01 0.01 0.01 0.00\r\n0.01 0.01 0.00 0.00\r\n0.01 0.01 0.01 0.00\r\n0.01 0.01 0.01 0.00\r\n0.01 0.01 0.00 0.00\r\n0.01 0.00 0.01 0.00\r\n0.01 0.01 0.01 0.00\r\n0.00 0.01 0.00 0.00\r\n0.01 0.01 0.01 0.00\r\n0.01 0.01 0.01 0.00\r\n0.00 0.01 0.00 0.00\r\n0.01 0.01 0.01 0.00\r\n0.01 0.01 0.01 0.00\r\n0.00 0.00 0.00 0.00\r\n0.01 0.01 0.00 0.00\r\n0.01 0.01 0.01 0.00\r\n0.01 0.01 0.01 0.00\r\n0.00 0.01 0.00 0.00\r\n0.01 0.01 0.01 0.00\r\n0.01 0.00 0.01 0.00\r\n0.00 0.01 0.01 0.00\r\n0.01 0.01 0.01 0.00\r\n0.00 0.01 0.01 0.00\r\n0.01 0.01 0.01 0.00\r\n0.01 0.01 0.01 0.00\r\n0.00 0.01 0.00 0.00\r\n0.00 0.00 0.01 0.00\r\n0.01 0.01 0.01 0.00\r\n0.01 0.01 0.01 0.00\r\n0.01 0.01 0.01 0.00\r\n0.01 0.01 0.01 0.00\r\n0.01 0.01 0.01 0.00\r\n0.01 0.01 0.01 0.00\r\n0.01 0.01 0.01 0.00\r\n0.00 0.01 0.01 0.00\r\n0.01 0.01 0.01 0.00\r\n0.01 0.01 0.01 0.00\r\n0.01 0.01 0.01 0.00\r\n0.01 0.01 0.01 0.00\r\n0.01 0.01 0.01 0.00\r\n0.00 0.01 0.01 0.00\r\n0.01 0.00 0.01 0.00\r\n0.01 0.01 0.01 0.00\r\n0.01 0.01 0.00 0.00\r\n0.00 0.01 0.00 0.00\r\n0.01 0.01 0.01 0.00\r\n0.01 0.01 0.01 0.00\r\n0.01 0.00 0.00 0.00\r\n0.00 0.01 0.01 0.00\r\n0.01 0.01 0.01 0.00\r\n0.01 0.01 0.01 0.00\r\n0.01 0.01 0.01 0.00\r\n0.01 0.02 0.01 0.00\r\n0.01 0.00 0.00 0.00\r\n0.00 0.00 0.00 0.00\r\n0.00 0.01 0.01 0.00\r\n0.01 0.01 0.01 0.00\r\n0.01 0.01 0.01 0.00\r\n0.01 0.01 0.01 0.00\r\n0.01 0.01 0.00 0.00\r\n0.01 0.01 0.01 0.00\r\n0.01 0.00 0.00 0.00\r\n0.00 0.01 0.00 0.00\r\n0.01 0.01 0.01 0.00\r\n0.01 0.01 0.01 0.00\r\n0.01 0.01 0.01 0.00\r\n0.01 0.00 0.01 0.00\r\n0.01 0.01 0.01 0.00\r\n0.01 0.01 0.01 0.00\r\n0.01 0.01 0.01 0.00\r\n0.01 0.01 0.01 0.00\r\n0.01 0.01 0.01 0.00\r\n0.00 0.00 0.01 0.00\r\n0.01 0.01 0.01 0.00\r\n0.01 0.01 0.01 0.00\r\n0.01 0.01 0.01 0.00\r\n0.01 0.01 0.01 0.00\r\n0.00 0.01 0.01 0.00\r\n0.00 0.01 0.00 0.00\r\n0.01 0.01 0.01 0.00\r\n0.01 0.01 0.01 0.00\r\n0.00 0.00 0.01 0.00\r\n0.00 0.00 0.00 0.00\r\n0.01 0.01 0.01 0.00\r\n0.00 0.01 0.01 0.00\r\n0.01 0.01 0.01 0.00\r\n0.00 0.01 0.01 0.00\r\n0.01 0.01 0.01 0.00\r\n0.01 0.01 0.01 0.00\r\n0.01 0.00 0.00 0.00\r\n0.01 0.01 0.00 0.00\r\n0.00 0.00 0.00 0.00\r\n0.01 0.00 0.01 0.00\r\n0.01 0.00 0.00 0.00\r\n0.01 0.02 0.01 0.00\r\n0.01 0.00 0.00 0.00\r\n0.00 0.00 0.01 0.00\r\n0.01 0.01 0.01 0.00\r\n0.01 0.01 0.01 0.00\r\n0.01 0.01 0.00 0.00\r\n0.01 0.01 0.01 0.00\r\n0.01 0.00 0.01 0.00\r\n0.01 0.00 0.01 0.00\r\n0.01 0.00 0.01 0.00\r\n0.01 0.01 0.01 0.00\r\n0.01 0.00 0.01 0.00\r\n0.01 0.01 0.01 0.00\r\n0.01 0.01 0.01 0.00\r\n0.00 0.01 0.00 0.00\r\n0.01 0.01 0.01 0.00\r\n0.01 0.01 0.01 0.00\r\n0.00 0.01 0.01 0.00\r\n0.00 0.00 0.00 0.00\r\n0.01 0.01 0.01 0.00\r\n0.00 0.00 0.01 0.00\r\n0.01 0.01 0.01 0.00\r\n0.01 0.01 0.00 0.00\r\n0.01 0.01 0.00 0.00\r\n0.01 0.01 0.01 0.00\r\n0.01 0.02 0.01 0.00\r\n0.01 0.01 0.00 0.00\r\n0.01 0.01 0.01 0.00\r\n0.01 0.01 0.01 0.00\r\n0.01 0.00 0.01 0.00\r\n0.01 -0.00 0.01 0.00\r\n0.01 0.01 0.01 0.00\r\n0.01 0.01 0.01 0.00\r\n0.01 0.01 0.01 0.00\r\n0.00 0.01 0.01 0.00\r\n0.01 0.01 0.01 0.00\r\n0.00 -0.00 0.00 0.00\r\n0.00 0.01 0.01 0.00\r\n0.01 0.01 0.02 0.00\r\n0.00 0.01 0.01 0.00\r\n0.00 0.01 0.01 0.00\r\n0.01 0.01 0.01 0.00\r\n0.01 0.01 0.01 0.00\r\n0.01 0.01 0.01 0.00\r\n0.01 0.00 0.01 0.00\r\n0.01 0.01 0.00 0.00\r\n0.00 0.01 0.01 0.00\r\n0.01 0.01 0.01 0.00\r\n0.01 0.01 0.01 0.00\r\n0.00 0.00 0.00 0.00\r\n0.01 0.01 0.01 0.00\r\n0.00 0.00 0.01 0.00\r\n0.01 0.00 0.00 0.00\r\n0.01 0.01 0.00 0.00\r\n0.00 0.01 0.01 0.00\r\n-0.00 0.01 0.01 0.00\r\n0.01 0.01 0.00 0.00\r\n0.00 0.01 0.00 0.00\r\n0.00 0.01 0.00 0.00\r\n0.01 0.01 0.01 0.00\r\n0.01 0.01 0.01 0.00\r\n0.01 0.00 0.00 0.00\r\n0.01 0.01 0.01 0.00\r\n0.00 0.00 0.01 0.00\r\n0.01 0.01 0.01 0.00\r\n0.01 0.01 0.01 0.00\r\n0.01 0.01 0.01 0.00\r\n0.01 0.01 0.01 0.00\r\n0.00 0.01 0.01 0.00\r\n0.01 0.01 0.00 0.00\r\n0.01 0.01 0.01 0.00\r\n0.01 0.01 0.01 0.00\r\n0.01 0.01 0.01 0.00\r\n0.01 0.00 0.00 0.00\r\n0.00 0.01 0.01 0.00\r\n0.01 0.01 0.01 0.00\r\n0.01 0.01 0.00 0.00\r\n0.02 0.01 0.01 0.00\r\n0.01 0.01 0.01 0.00\r\n0.01 0.00 0.01 0.00\r\n0.01 0.01 0.00 0.00\r\n0.00 0.01 0.01 0.00\r\n0.01 0.01 0.01 0.00\r\n0.01 0.01 0.00 0.00\r\n0.01 0.01 0.01 0.00\r\n0.00 0.01 0.01 0.00\r\n0.01 0.01 0.00 0.00\r\n0.01 0.01 0.01 0.00\r\n0.01 0.02 0.01 0.00\r\n0.00 0.01 0.01 0.00\r\n0.01 0.00 0.01 0.00\r\n0.00 0.01 0.00 0.00\r\n0.00 0.01 0.01 0.00\r\n0.02 0.01 0.01 0.00\r\n0.01 0.01 0.01 0.00\r\n0.01 0.01 0.01 0.00\r\n0.01 0.00 0.01 0.00\r\n0.00 0.01 0.00 0.00\r\n0.01 0.01 0.01 0.00\r\n0.01 0.00 0.01 0.00\r\n0.01 0.01 0.00 0.00\r\n0.01 0.01 0.01 0.00\r\n0.01 0.01 0.01 0.00\r\n0.01 0.01 0.01 0.00\r\n0.00 0.01 0.01 0.00\r\n0.01 0.01 0.01 0.00\r\n0.01 0.01 0.01 0.00\r\n0.01 0.01 0.01 0.00\r\n0.01 0.01 0.01 0.00\r\n0.00 0.00 -0.00 0.00\r\n0.01 0.00 0.01 0.00\r\n0.01 0.01 0.01 0.00\r\n0.01 0.00 0.01 0.00\r\n0.01 0.01 0.01 0.00\r\n0.01 0.00 0.00 0.00\r\n0.01 0.01 0.01 0.00\r\n0.01 0.01 0.00 0.00\r\n0.01 0.01 0.01 0.00\r\n0.02 0.00 0.01 0.00\r\n0.01 0.00 0.00 0.00\r\n0.00 0.01 0.00 0.00\r\n-0.00 0.00 -0.00 0.00\r\n0.01 0.01 0.01 0.00\r\n0.01 0.00 0.01 0.00\r\n0.00 0.00 0.01 0.00\r\n0.00 0.00 0.01 0.00\r\n-0.01 -0.00 0.00 0.00\r\n0.01 -0.00 -0.00 0.00\r\n-0.00 -0.00 -0.00 0.00\r\n-0.00 0.00 0.01 0.00\r\n0.00 0.00 0.00 0.00\r\n-0.00 -0.00 -0.00 0.00\r\n-0.00 0.00 0.00 0.00\r\n0.00 0.00 0.00 0.00\r\n0.00 -0.00 0.00 0.00\r\n0.00 0.00 0.00 0.00\r\n0.01 0.00 0.01 0.00\r\n-0.00 -0.00 -0.00 0.00\r\n0.00 0.00 0.01 0.00\r\n0.00 0.00 0.01 0.00\r\n0.01 0.01 0.01 0.00\r\n0.00 0.01 0.01 0.00\r\n0.00 0.00 0.00 0.00\r\n-0.00 0.00 -0.01 0.00\r\n0.01 0.01 0.00 0.00\r\n0.01 0.01 0.01 0.00\r\n0.00 0.01 0.01 0.00\r\n0.00 0.01 0.01 0.00\r\n0.00 0.01 0.01 0.00\r\n0.00 0.00 0.01 0.00\r\n0.01 0.01 0.01 0.00\r\n0.01 0.01 0.01 0.00\r\n0.01 0.01 0.01 0.00\r\n0.01 0.01 0.01 0.00\r\n0.00 0.01 0.01 0.00\r\n0.00 0.01 0.01 0.00\r\n0.01 0.01 0.00 0.00\r\n0.01 -0.00 0.00 0.00\r\n0.01 0.01 0.00 0.00\r\n-0.00 0.01 0.01 0.00\r\n0.01 0.01 0.01 0.00\r\n0.01 0.00 0.01 0.00\r\n0.01 0.01 0.01 0.00\r\n0.00 0.01 0.01 0.00\r\n0.01 0.00 0.01 0.00\r\n0.01 0.01 0.01 0.00\r\n0.00 -0.00 0.00 0.00\r\n0.01 0.01 0.01 0.00\r\n0.01 0.01 0.01 0.00\r\n0.01 0.01 0.01 0.00\r\n0.02 0.00 0.01 0.00\r\n0.01 0.01 0.01 0.00\r\n0.01 0.01 0.00 0.00\r\n0.01 0.01 0.02 0.00\r\n0.01 0.01 0.01 0.00\r\n0.01 0.01 0.01 0.00\r\n0.00 0.01 0.00 0.00\r\n0.01 0.01 0.00 0.00\r\n0.00 0.00 0.01 0.00\r\n0.01 0.01 0.01 0.00\r\n0.01 0.01 0.01 0.00\r\n0.01 0.01 0.01 0.00\r\n0.01 0.01 0.01 0.00\r\n0.02 0.01 0.01 0.00\r\n0.00 0.01 0.01 0.00\r\n0.01 0.00 0.00 0.00\r\n0.01 0.01 0.01 0.00\r\n0.01 0.01 0.01 0.00\r\n0.01 0.00 0.01 0.00\r\n0.01 0.01 0.01 0.00\r\n0.01 0.01 0.01 0.00\r\n0.01 0.01 0.01 0.00\r\n0.01 0.01 0.01 0.00\r\n0.01 0.01 0.01 0.00\r\n0.01 0.01 0.00 0.00\r\n0.01 0.00 0.01 0.00\r\n0.01 0.01 0.01 0.00\r\n0.01 0.01 0.01 0.00\r\n0.01 0.01 0.01 0.00\r\n0.01 0.00 0.01 0.00\r\n0.01 0.01 0.01 0.00\r\n0.01 0.01 0.01 0.00\r\n0.01 0.01 0.01 0.00\r\n0.02 0.01 0.01 0.00\r\n0.01 0.01 0.01 0.00\r\n0.01 0.00 0.01 0.00\r\n0.01 0.01 0.01 0.00\r\n0.01 0.00 0.00 0.00\r\n0.01 0.01 0.01 0.00\r\n0.00 0.01 0.01 0.00\r\n0.01 0.01 0.00 0.00\r\n0.01 0.01 0.01 0.00\r\n0.01 0.01 0.01 0.00\r\n0.01 0.01 0.01 0.00\r\n0.00 0.00 0.00 0.00\r\n0.01 0.01 0.01 0.00\r\n0.01 0.01 0.00 0.00\r\n0.00 0.01 0.00 0.00\r\n0.01 0.00 0.00 0.00\r\n0.00 0.01 0.01 0.00\r\n0.01 0.01 0.00 0.00\r\n0.00 0.00 0.01 0.00\r\n0.01 0.01 0.01 0.00\r\n0.01 0.00 0.00 0.00\r\n0.00 0.01 0.00 0.00\r\n0.01 0.02 0.01 0.00\r\n0.01 0.01 0.00 0.00\r\n0.01 0.01 0.01 0.00\r\n0.01 0.01 0.01 0.00\r\n0.01 0.00 0.01 0.00\r\n0.01 0.01 0.01 0.00\r\n0.01 0.01 0.01 0.00\r\n0.00 -0.00 -0.00 0.00\r\n0.01 0.01 0.01 0.00\r\n0.01 0.01 0.01 0.00\r\n0.00 0.01 0.01 0.00\r\n0.01 0.01 0.01 0.00\r\n0.01 0.01 0.01 0.00\r\n0.00 0.01 0.01 0.00\r\n0.01 0.01 0.01 0.00\r\n0.01 0.01 0.00 0.00\r\n0.01 0.01 0.01 0.00\r\n0.00 0.00 -0.00 0.00\r\n0.01 0.01 0.01 0.00\r\n0.01 0.01 0.01 0.00\r\n0.01 0.01 0.00 0.00\r\n0.01 0.01 0.01 0.00\r\n0.01 0.01 0.01 0.00\r\n0.00 0.01 0.01 0.00\r\n0.00 0.01 0.01 0.00\r\n0.01 0.01 0.01 0.00\r\n0.01 0.00 0.00 0.00\r\n0.00 0.01 0.00 0.00\r\n0.00 0.01 0.00 0.00\r\n0.00 0.01 0.01 0.00\r\n0.00 0.01 0.00 0.00\r\n0.01 0.00 0.01 0.00\r\n0.00 0.01 0.01 0.00\r\n0.01 0.01 0.01 0.00\r\n0.01 0.00 0.01 0.00\r\n0.00 0.01 0.01 0.00\r\n-0.01 0.01 0.00 0.00\r\n0.01 0.01 0.00 0.00\r\n0.00 0.00 0.00 0.00\r\n0.00 0.01 0.01 0.00\r\n0.00 -0.00 0.01 0.00\r\n0.01 0.01 0.00 0.00\r\n0.01 0.01 0.01 0.00\r\n0.00 0.01 0.01 0.00\r\n0.00 0.00 0.01 0.00\r\n0.00 0.00 0.00 0.00\r\n0.01 -0.00 0.01 0.00\r\n0.00 0.00 0.01 0.00\r\n0.00 0.01 0.01 0.00\r\n0.01 0.01 0.01 0.00\r\n0.00 0.01 0.01 0.00\r\n0.00 0.01 0.00 0.00\r\n0.00 0.00 0.00 0.00\r\n-0.00 0.01 0.01 0.00\r\n0.00 0.01 0.01 0.00\r\n0.00 0.01 0.01 0.00\r\n0.01 0.00 0.01 0.00\r\n0.01 0.00 0.00 0.00\r\n0.01 0.00 0.01 0.00\r\n0.01 0.00 0.01 0.00\r\n0.01 0.01 0.01 0.00\r\n0.01 0.01 0.01 0.00\r\n0.01 0.00 0.01 0.00\r\n0.01 0.01 0.00 0.00\r\n0.01 0.01 0.01 0.00\r\n0.01 0.01 0.01 0.00\r\n0.01 0.01 0.01 0.00\r\n0.01 0.01 0.00 0.00\r\n0.01 0.01 0.01 0.00\r\n0.01 0.00 0.00 0.00\r\n0.01 0.01 0.01 0.00\r\n0.02 0.01 0.01 0.00\r\n0.01 0.01 0.01 0.00\r\n0.01 0.01 0.01 0.00\r\n0.01 0.01 0.01 0.00\r\n0.00 0.00 0.00 0.00\r\n0.01 0.01 0.01 0.00\r\n0.01 0.00 0.00 0.00\r\n0.01 0.00 0.01 0.00\r\n0.01 0.01 0.00 0.00\r\n0.01 0.01 0.01 0.00\r\n0.01 0.01 0.01 0.00\r\n0.02 0.01 0.02 0.00\r\n0.01 0.01 0.01 0.00\r\n0.01 0.01 0.01 0.00\r\n0.01 0.01 0.01 0.00\r\n0.01 0.01 0.01 0.00\r\n0.00 0.01 0.01 0.00\r\n0.02 0.01 0.01 0.00\r\n0.01 0.01 0.01 0.00\r\n0.01 0.01 0.01 0.00\r\n0.01 0.01 0.01 0.00\r\n0.01 0.01 0.02 0.00\r\n0.02 0.02 0.02 0.00\r\n0.01 0.01 0.00 0.00\r\n0.01 0.01 0.01 0.00\r\n0.02 0.01 0.01 0.00\r\n0.01 0.01 0.01 0.00\r\n0.01 0.01 0.01 0.00\r\n0.01 0.01 0.01 0.00\r\n0.01 0.01 0.01 0.00\r\n0.01 0.01 0.02 0.00\r\n0.01 0.01 0.01 0.00\r\n0.00 0.01 0.01 0.00\r\n0.01 0.01 0.02 0.00\r\n0.01 0.01 0.01 0.00\r\n0.01 0.01 0.01 0.00\r\n0.00 0.01 0.01 0.00\r\n0.01 0.00 0.01 0.00\r\n0.00 0.01 0.01 0.00\r\n0.01 0.01 0.01 0.00\r\n0.01 0.01 0.01 0.00\r\n0.00 0.01 0.01 0.00\r\n0.00 0.01 0.01 0.00\r\n0.01 0.00 0.01 0.00\r\n0.01 0.01 0.01 0.00\r\n0.01 0.00 0.01 0.00\r\n0.01 0.01 0.01 0.00\r\n0.01 0.01 0.00 0.00\r\n0.00 0.01 0.00 0.00\r\n0.01 0.00 0.01 0.00\r\n0.01 0.01 0.01 0.00\r\n0.01 0.01 0.01 0.00\r\n0.01 0.01 0.01 0.00\r\n0.00 0.00 0.01 0.00\r\n0.01 0.01 0.00 0.00\r\n0.01 0.01 0.01 0.00\r\n0.00 0.01 0.01 0.00\r\n0.00 0.00 0.00 0.00\r\n0.01 0.01 0.01 0.00\r\n0.01 0.00 0.01 0.00\r\n0.01 0.01 0.01 0.00\r\n0.00 0.01 0.00 0.00\r\n0.01 0.00 0.00 0.00\r\n0.01 0.00 0.01 0.00\r\n0.00 0.00 0.00 0.00\r\n0.01 0.00 0.01 0.00\r\n0.01 0.01 0.01 0.00\r\n0.01 0.01 0.02 0.00\r\n0.01 0.01 0.00 0.00\r\n0.01 0.00 0.00 0.00\r\n0.01 0.01 0.00 0.00\r\n0.01 0.00 0.01 0.00\r\n0.00 0.01 0.01 0.00\r\n0.01 0.01 0.01 0.00\r\n0.01 0.01 0.01 0.00\r\n0.01 0.01 0.00 0.00\r\n0.01 0.01 0.01 0.00\r\n0.01 0.01 0.01 0.00\r\n0.01 0.01 0.01 0.00\r\n0.00 0.01 0.00 0.00\r\n0.01 0.01 0.01 0.00\r\n0.01 0.01 0.01 0.00\r\n0.01 0.01 0.01 0.00\r\n0.01 0.00 0.02 0.00\r\n0.01 0.01 0.01 0.00\r\n0.01 0.01 0.01 0.00\r\n0.01 0.01 0.01 0.00\r\n0.01 0.01 0.01 0.00\r\n0.00 0.01 0.01 0.00\r\n0.00 0.01 0.01 0.00\r\n0.00 0.01 0.00 0.00\r\n0.00 0.01 0.01 0.00\r\n0.01 0.01 0.01 0.00\r\n0.01 0.01 0.00 0.00\r\n0.01 0.01 0.01 0.00\r\n0.01 0.02 0.01 0.00\r\n0.01 0.01 0.00 0.00\r\n0.01 0.01 0.01 0.00\r\n0.01 0.01 0.01 0.00\r\n0.01 0.01 0.01 0.00\r\n0.01 0.00 0.00 0.00\r\n0.01 0.01 0.01 0.00\r\n0.00 0.00 0.00 0.00\r\n0.01 0.01 0.01 0.00\r\n0.00 0.01 0.01 0.00\r\n0.01 0.01 0.01 0.00\r\n0.00 0.01 0.00 0.00\r\n0.00 0.01 0.01 0.00\r\n0.00 0.01 0.00 0.00\r\n0.01 0.02 0.01 0.00\r\n0.00 0.01 0.00 0.00\r\n0.01 0.00 0.01 0.00\r\n0.01 0.00 0.01 0.00\r\n0.01 0.00 0.00 0.00\r\n0.00 0.01 0.01 0.00\r\n0.00 0.01 0.00 0.00\r\n0.00 0.01 0.01 0.00\r\n0.01 0.01 0.02 0.00\r\n0.01 -0.00 0.00 0.00\r\n0.01 0.01 0.01 0.00\r\n0.01 0.01 0.01 0.00\r\n0.01 0.01 0.00 0.00\r\n0.01 0.01 0.01 0.00\r\n0.01 0.00 0.00 0.00\r\n0.00 0.01 0.00 0.00\r\n0.00 0.01 0.01 0.00\r\n0.01 -0.00 0.01 0.00\r\n0.01 0.00 0.01 0.00\r\n0.01 0.01 0.01 0.00\r\n0.01 0.00 0.01 0.00\r\n0.01 0.01 0.00 0.00\r\n0.00 0.01 0.01 0.00\r\n0.01 0.01 0.00 0.00\r\n0.01 0.01 0.01 0.00\r\n0.01 0.01 0.01 0.00\r\n0.01 0.01 0.01 0.00\r\n0.01 0.01 0.01 0.00\r\n0.01 0.01 0.01 0.00\r\n0.01 0.01 0.01 0.00\r\n0.01 0.01 0.01 0.00\r\n0.01 0.01 0.01 0.00\r\n0.01 0.01 0.01 0.00\r\n0.01 0.01 0.00 0.00\r\n0.01 0.01 0.01 0.00\r\n0.01 0.01 0.01 0.00\r\n0.01 0.01 0.01 0.00\r\n0.01 0.01 0.02 0.00\r\n0.01 0.01 0.01 0.00\r\n0.01 0.00 0.01 0.00\r\n-0.00 0.01 0.01 0.00\r\n0.01 0.01 0.01 0.00\r\n0.01 0.01 0.01 0.00\r\n0.01 0.00 -0.00 0.00\r\n0.00 0.01 0.01 0.00\r\n0.01 0.01 0.01 0.00\r\n0.01 0.00 0.01 0.00\r\n0.01 0.01 0.01 0.00\r\n0.02 0.01 0.02 0.00\r\n0.00 0.01 0.01 0.00\r\n0.01 0.01 0.01 0.00\r\n0.01 0.00 0.01 0.00\r\n0.01 0.00 0.00 0.00\r\n0.01 0.01 0.00 0.00\r\n0.00 0.01 0.01 0.00\r\n0.00 0.01 0.00 0.00\r\n0.00 0.00 0.01 0.00\r\n0.01 0.01 0.00 0.00\r\n0.01 0.00 0.00 0.00\r\n0.01 0.01 0.00 0.00\r\n0.00 0.00 -0.00 0.00\r\n0.01 0.00 0.00 0.00\r\n-0.00 -0.00 -0.00 0.00\r\n0.01 0.01 0.01 0.00\r\n0.00 0.01 0.01 0.00\r\n0.01 0.01 0.01 0.00\r\n0.00 0.01 0.00 0.00\r\n0.00 0.00 0.01 0.00\r\n0.00 0.00 0.00 0.00\r\n0.00 0.01 0.01 0.00\r\n0.01 0.00 0.01 0.00\r\n0.01 0.01 0.01 0.00\r\n0.01 0.00 0.00 0.00\r\n0.01 0.01 0.00 0.00\r\n0.00 0.00 0.01 0.00\r\n0.01 0.00 0.01 0.00\r\n0.01 0.00 0.01 0.00\r\n0.00 0.01 0.00 0.00\r\n0.01 0.01 0.01 0.00\r\n-0.00 0.00 0.00 0.00\r\n0.01 0.00 0.00 0.00\r\n0.01 0.01 0.01 0.00\r\n0.01 0.00 0.01 0.00\r\n-0.00 0.01 0.00 0.00\r\n0.01 0.01 0.01 0.00\r\n0.01 0.00 0.01 0.00\r\n0.00 0.01 0.01 0.00\r\n0.00 0.01 0.01 0.00\r\n0.01 -0.00 0.00 0.00\r\n0.01 0.01 0.01 0.00\r\n0.01 0.01 0.01 0.00\r\n0.01 0.01 0.01 0.00\r\n0.01 0.01 0.00 0.00\r\n0.01 0.01 0.01 0.00\r\n0.01 0.01 0.01 0.00\r\n0.01 0.01 0.01 0.00\r\n0.01 0.01 0.01 0.00\r\n0.01 0.01 0.01 0.00\r\n0.01 0.01 0.01 0.00\r\n0.01 0.01 0.01 0.00\r\n0.02 0.01 0.02 0.00\r\n0.01 0.01 0.01 0.00\r\n0.01 0.01 0.01 0.00\r\n0.02 0.01 0.01 0.00\r\n0.01 0.01 0.01 0.00\r\n0.01 0.01 0.01 0.00\r\n0.01 0.01 0.01 0.00\r\n0.01 0.01 0.01 0.00\r\n0.01 0.01 0.01 0.00\r\n0.01 0.01 0.01 0.00\r\n0.02 0.01 0.02 0.00\r\n0.01 0.01 0.01 0.00\r\n0.01 0.01 0.02 0.00\r\n0.02 0.01 0.02 0.00\r\n0.01 0.01 0.01 0.00\r\n0.01 0.01 0.01 0.00\r\n0.01 0.01 0.01 0.00\r\n0.00 0.01 0.01 0.00\r\n0.01 0.01 0.01 0.00\r\n0.01 0.01 0.01 0.00\r\n0.01 0.01 0.01 0.00\r\n0.01 0.01 0.01 0.00\r\n0.02 0.01 0.01 0.00\r\n0.01 0.01 0.00 0.00\r\n0.01 0.01 0.01 0.00\r\n0.00 0.01 0.00 0.00\r\n0.01 0.01 0.01 0.00\r\n0.01 0.01 0.01 0.00\r\n0.01 0.01 0.01 0.00\r\n0.01 0.01 0.01 0.00\r\n0.01 0.01 0.01 0.00\r\n0.00 0.00 0.00 0.00\r\n0.00 -0.00 -0.00 0.00\r\n0.01 0.01 0.01 0.00\r\n0.01 0.00 0.01 0.00\r\n0.01 0.01 0.00 0.00\r\n0.01 0.02 0.01 0.00\r\n0.01 0.01 0.01 0.00\r\n0.01 0.01 0.02 0.00\r\n0.01 0.01 0.01 0.00\r\n0.01 0.01 0.00 0.00\r\n0.01 0.00 0.01 0.00\r\n0.01 0.01 0.00 0.00\r\n0.01 0.01 0.01 0.00\r\n0.01 0.01 0.01 0.00\r\n0.00 0.01 0.00 0.00\r\n0.00 0.01 0.01 0.00\r\n0.01 0.01 0.01 0.00\r\n0.00 0.01 0.01 0.00\r\n0.01 0.01 0.01 0.00\r\n0.01 0.01 0.01 0.00\r\n0.01 0.01 0.01 0.00\r\n0.01 0.01 0.01 0.00\r\n0.00 0.01 0.01 0.00\r\n0.00 0.01 0.00 0.00\r\n0.01 0.01 0.01 0.00\r\n0.00 0.00 0.01 0.00\r\n0.00 0.01 0.01 0.00\r\n0.00 0.02 0.01 0.00\r\n0.01 0.00 0.01 0.00\r\n0.01 0.01 0.01 0.00\r\n0.02 0.01 0.01 0.00\r\n0.01 0.01 0.02 0.00\r\n0.01 0.01 0.01 0.00\r\n0.01 0.01 0.01 0.00\r\n0.01 0.01 0.01 0.00\r\n0.01 0.01 0.01 0.00\r\n0.01 0.01 0.01 0.00\r\n0.01 0.00 0.01 0.00\r\n0.01 0.01 0.01 0.00\r\n0.01 0.01 0.01 0.00\r\n0.01 0.01 0.01 0.00\r\n0.01 0.01 0.01 0.00\r\n0.01 0.02 0.02 0.00\r\n0.01 0.01 0.01 0.00\r\n0.01 0.01 0.01 0.00\r\n0.01 0.02 0.01 0.00\r\n0.01 0.01 0.01 0.00\r\n0.01 0.01 0.01 0.00\r\n0.00 0.01 0.01 0.00\r\n0.01 0.01 0.01 0.00\r\n0.00 0.01 0.01 0.00\r\n0.00 0.01 0.00 0.00\r\n0.01 0.01 0.01 0.00\r\n0.01 0.01 0.01 0.00\r\n0.01 0.00 0.01 0.00\r\n0.01 0.01 0.01 0.00\r\n0.00 0.01 0.00 0.00\r\n0.00 0.01 0.00 0.00\r\n0.01 0.01 0.00 0.00\r\n-0.00 0.00 0.00 0.00\r\n0.00 0.01 0.01 0.00\r\n0.00 0.01 0.01 0.00\r\n0.00 0.01 0.01 0.00\r\n0.01 0.01 0.01 0.00\r\n0.01 0.01 0.01 0.00\r\n0.01 0.00 0.00 0.00\r\n0.01 0.01 0.01 0.00\r\n0.01 0.01 0.01 0.00\r\n0.01 0.01 0.01 0.00\r\n0.00 0.00 0.00 0.00\r\n0.01 0.01 0.01 0.00\r\n0.01 0.00 0.01 0.00\r\n0.01 0.00 0.01 0.00\r\n0.01 0.01 0.00 0.00\r\n0.00 0.00 0.00 0.00\r\n0.01 0.01 0.01 0.00\r\n0.01 0.00 -0.00 0.00\r\n0.01 0.00 0.00 0.00\r\n0.01 0.01 0.00 0.00\r\n0.01 0.00 0.01 0.00\r\n0.00 0.00 0.00 0.00\r\n0.01 0.01 0.01 0.00\r\n0.00 0.01 0.00 0.00\r\n0.01 0.01 0.00 0.00\r\n0.00 0.00 0.01 0.00\r\n0.00 0.00 0.01 0.00\r\n0.01 0.01 0.01 0.00\r\n0.01 0.00 0.01 0.00\r\n0.00 0.01 0.00 0.00\r\n0.01 0.00 0.01 0.00\r\n0.01 0.01 0.01 0.00\r\n0.01 0.01 0.01 0.00\r\n0.01 0.01 0.01 0.00\r\n0.01 -0.00 0.01 0.00\r\n0.01 0.00 0.00 0.00\r\n0.01 0.00 0.01 0.00\r\n0.01 0.01 0.01 0.00\r\n0.00 0.01 0.00 0.00\r\n0.01 0.00 0.01 0.00\r\n0.00 0.01 0.01 0.00\r\n0.00 0.01 0.01 0.00\r\n0.00 0.01 0.00 0.00\r\n0.01 0.00 0.01 0.00\r\n0.00 0.01 0.01 0.00\r\n0.00 0.01 -0.00 0.00\r\n0.01 0.01 -0.00 0.00\r\n0.01 0.01 0.00 0.00\r\n0.01 0.01 0.01 0.00\r\n0.01 -0.00 0.00 0.00\r\n0.00 0.01 0.00 0.00\r\n0.01 0.01 0.01 0.00\r\n0.01 0.01 0.01 0.00\r\n0.01 0.00 0.00 0.00\r\n0.01 0.00 0.00 0.00\r\n0.01 0.00 0.00 0.00\r\n0.01 0.01 0.01 0.00\r\n0.00 0.01 0.01 0.00\r\n0.00 0.00 0.00 0.00\r\n0.00 0.01 0.00 0.00\r\n0.00 0.01 0.01 0.00\r\n0.01 0.00 0.00 0.00\r\n0.00 0.00 0.00 0.00\r\n0.00 0.00 0.00 0.00\r\n0.00 0.01 0.01 0.00\r\n0.01 0.01 0.01 0.00\r\n0.02 0.00 0.01 0.00\r\n0.01 0.01 0.00 0.00\r\n0.01 0.01 0.01 0.00\r\n0.01 0.01 0.01 0.00\r\n0.01 0.01 0.02 0.00\r\n0.01 0.01 0.01 0.00\r\n0.01 0.01 0.00 0.00\r\n0.01 0.01 0.01 0.00\r\n0.00 0.01 0.01 0.00\r\n0.01 0.02 0.01 0.00\r\n0.01 -0.00 0.00 0.00\r\n0.01 -0.00 0.00 0.00\r\n0.01 0.01 0.01 0.00\r\n0.01 0.01 0.01 0.00\r\n0.01 0.01 0.01 0.00\r\n0.01 0.01 0.01 0.00\r\n0.01 0.01 0.01 0.00\r\n0.01 0.01 0.01 0.00\r\n0.01 0.01 0.01 0.00\r\n0.01 0.00 0.01 0.00\r\n0.01 0.01 0.01 0.00\r\n0.01 0.00 0.00 0.00\r\n0.01 0.01 0.01 0.00\r\n0.01 0.01 0.01 0.00\r\n-0.00 0.01 0.01 0.00\r\n0.01 0.01 0.00 0.00\r\n0.01 0.00 0.01 0.00\r\n0.00 0.00 0.01 0.00\r\n0.00 0.01 0.01 0.00\r\n0.01 0.01 0.01 0.00\r\n0.01 0.01 0.01 0.00\r\n0.01 0.01 0.01 0.00\r\n0.01 0.01 0.01 0.00\r\n0.00 0.00 0.01 0.00\r\n0.01 0.01 0.02 0.00\r\n0.01 0.00 0.00 0.00\r\n0.00 0.01 0.00 0.00\r\n0.00 0.00 0.01 0.00\r\n0.01 0.01 0.01 0.00\r\n0.01 0.00 0.00 0.00\r\n0.01 0.01 0.01 0.00\r\n0.01 0.01 0.01 0.00\r\n0.01 0.01 0.00 0.00\r\n0.00 0.01 0.00 0.00\r\n0.01 0.00 0.01 0.00\r\n0.01 0.01 0.01 0.00\r\n0.01 0.01 0.01 0.00\r\n0.01 0.01 0.00 0.00\r\n0.01 0.01 0.01 0.00\r\n0.01 0.01 0.01 0.00\r\n0.00 0.01 0.01 0.00\r\n0.01 0.01 0.01 0.00\r\n0.01 0.01 0.01 0.00\r\n0.00 0.01 0.01 0.00\r\n0.00 0.01 0.00 0.00\r\n0.00 0.01 0.01 0.00\r\n0.01 0.00 0.01 0.00\r\n0.01 0.01 0.01 0.00\r\n0.00 0.02 0.01 0.00\r\n0.01 0.02 0.02 0.00\r\n0.00 0.01 0.01 0.00\r\n0.00 0.01 0.01 0.00\r\n0.01 0.01 0.01 0.00\r\n0.01 0.00 0.01 0.00\r\n0.00 0.00 0.01 0.00\r\n0.01 0.01 0.01 0.00\r\n0.01 0.01 0.00 0.00\r\n0.01 0.01 0.00 0.00\r\n0.01 0.01 0.01 0.00\r\n0.01 0.01 0.01 0.00\r\n0.01 0.01 0.01 0.00\r\n0.01 0.01 0.01 0.00\r\n0.00 0.01 0.01 0.00\r\n0.00 0.00 0.00 0.00\r\n0.01 0.01 0.01 0.00\r\n0.01 0.00 0.01 0.00\r\n0.00 0.01 0.00 0.00\r\n0.01 0.01 0.01 0.00\r\n0.01 0.01 0.01 0.00\r\n0.01 0.01 0.00 0.00\r\n0.01 0.01 0.01 0.00\r\n0.01 0.00 0.00 0.00\r\n0.00 0.01 0.00 0.00\r\n0.01 0.00 0.01 0.00\r\n0.01 0.01 0.01 0.00\r\n0.01 0.00 0.00 0.00\r\n0.01 0.01 0.01 0.00\r\n0.01 0.01 0.01 0.00\r\n0.01 0.01 0.01 0.00\r\n0.01 0.01 0.01 0.00\r\n0.01 0.01 0.01 0.00\r\n0.00 0.01 0.00 0.00\r\n0.01 0.01 0.01 0.00\r\n0.01 0.01 0.00 0.00\r\n0.01 0.00 0.01 0.00\r\n0.01 0.01 0.01 0.00\r\n0.00 0.00 0.01 0.00\r\n0.01 0.01 0.01 0.00\r\n0.00 0.00 0.01 0.00\r\n0.01 0.00 0.01 0.00\r\n0.00 0.00 0.00 0.00\r\n0.01 0.00 0.01 0.00\r\n0.00 0.01 0.01 0.00\r\n0.00 0.01 -0.00 0.00\r\n0.00 0.01 0.00 0.00\r\n0.01 0.01 0.01 0.00\r\n0.00 0.01 0.01 0.00\r\n0.01 0.00 0.00 0.00\r\n0.01 0.01 0.01 0.00\r\n0.01 0.01 0.00 0.00\r\n0.01 0.01 0.01 0.00\r\n0.01 0.01 0.01 0.00\r\n0.01 0.01 0.01 0.00\r\n0.00 0.00 0.00 0.00\r\n0.01 0.01 0.01 0.00\r\n0.01 0.00 0.01 0.00\r\n0.01 0.01 0.01 0.00\r\n0.00 0.01 0.01 0.00\r\n0.01 0.00 0.01 0.00\r\n0.01 0.01 0.01 0.00\r\n0.00 0.01 0.01 0.00\r\n0.01 0.01 0.01 0.00\r\n0.01 0.01 0.01 0.00\r\n0.01 0.00 0.01 0.00\r\n0.01 0.00 0.01 0.00\r\n0.00 0.00 0.01 0.00\r\n0.00 0.01 0.00 0.00\r\n0.01 0.01 0.01 0.00\r\n0.00 0.00 0.00 0.00\r\n0.00 0.01 0.01 0.00\r\n0.01 0.01 0.01 0.00\r\n0.01 0.01 0.01 0.00\r\n0.01 0.01 0.00 0.00\r\n0.01 0.01 0.01 0.00\r\n0.01 0.01 0.00 0.00\r\n0.01 0.00 0.01 0.00\r\n0.01 0.01 0.01 0.00\r\n0.01 0.00 0.01 0.00\r\n0.00 0.01 0.01 0.00\r\n0.01 0.00 0.01 0.00\r\n0.01 0.00 0.01 0.00\r\n0.01 0.01 0.01 0.00\r\n0.02 0.01 0.01 0.00\r\n0.01 0.00 0.00 0.00\r\n0.01 0.01 0.01 0.00\r\n0.02 0.01 0.02 0.00\r\n0.01 0.00 0.00 0.00\r\n0.01 0.01 0.01 0.00\r\n0.01 0.00 0.00 0.00\r\n0.01 0.00 0.01 0.00\r\n0.01 0.01 0.00 0.00\r\n0.01 0.01 0.01 0.00\r\n0.00 0.01 0.00 0.00\r\n-0.00 0.00 0.00 0.00\r\n0.00 0.00 0.01 0.00\r\n0.02 0.01 0.01 0.00\r\n0.01 0.00 0.01 0.00\r\n0.00 0.01 0.01 0.00\r\n0.01 0.00 0.01 0.00\r\n0.00 0.00 0.00 0.00\r\n0.01 0.00 0.00 0.00\r\n0.00 0.01 0.00 0.00\r\n0.01 0.01 0.01 0.00\r\n0.01 0.01 0.01 0.00\r\n0.01 0.01 0.01 0.00\r\n0.01 0.00 0.01 0.00\r\n0.00 0.01 0.01 0.00\r\n0.01 0.00 0.01 0.00\r\n0.01 0.00 0.00 0.00\r\n0.01 0.00 0.01 0.00\r\n0.01 0.00 0.01 0.00\r\n0.01 0.01 0.01 0.00\r\n0.01 0.02 0.01 0.00\r\n0.01 0.01 0.01 0.00\r\n0.00 0.00 0.00 0.00\r\n0.00 0.01 0.01 0.00\r\n0.01 0.01 0.01 0.00\r\n0.00 0.01 0.01 0.00\r\n0.00 0.01 0.00 0.00\r\n0.00 -0.00 0.00 0.00\r\n0.01 0.00 0.00 0.00\r\n0.01 0.01 0.01 0.00\r\n0.01 0.00 0.01 0.00\r\n0.00 0.00 -0.00 0.00\r\n0.01 0.01 0.00 0.00\r\n0.01 0.02 0.01 0.00\r\n0.01 0.01 0.01 0.00\r\n0.01 0.01 0.01 0.00\r\n0.01 0.01 0.01 0.00\r\n0.01 0.01 0.01 0.00\r\n0.01 0.01 0.00 0.00\r\n0.01 0.01 0.01 0.00\r\n0.01 0.00 0.00 0.00\r\n0.01 0.00 0.01 0.00\r\n0.00 0.01 0.01 0.00\r\n0.00 0.01 0.01 0.00\r\n0.01 0.00 0.01 0.00\r\n0.00 0.01 0.01 0.00\r\n0.00 0.01 0.01 0.00\r\n0.01 0.01 0.01 0.00\r\n0.00 0.01 0.01 0.00\r\n0.01 0.01 0.01 0.00\r\n0.01 0.01 0.00 0.00\r\n0.01 0.01 0.01 0.00\r\n0.01 0.01 0.00 0.00\r\n0.00 0.01 0.01 0.00\r\n0.01 0.00 0.01 0.00\r\n0.01 0.00 0.01 0.00\r\n0.01 0.00 0.00 0.00\r\n0.00 0.01 0.00 0.00\r\n0.01 0.01 0.01 0.00\r\n0.00 0.01 0.01 0.00\r\n0.00 0.01 0.01 0.00\r\n0.01 0.01 0.01 0.00\r\n0.00 0.00 0.00 0.00\r\n0.01 0.01 0.01 0.00\r\n0.01 0.00 0.00 0.00\r\n0.00 0.01 0.01 0.00\r\n0.01 0.01 0.01 0.00\r\n0.01 0.01 0.02 0.00\r\n0.01 0.01 0.01 0.00\r\n0.01 0.01 0.01 0.00\r\n0.01 0.01 0.01 0.00\r\n0.00 0.01 0.00 0.00\r\n0.01 0.00 0.01 0.00\r\n0.01 0.00 0.01 0.00\r\n0.01 0.00 0.00 0.00\r\n0.01 0.01 0.01 0.00\r\n0.00 0.01 0.01 0.00\r\n0.01 0.01 0.01 0.00\r\n0.01 0.01 0.00 0.00\r\n0.01 0.01 0.01 0.00\r\n0.01 0.00 0.01 0.00\r\n0.00 0.01 0.01 0.00\r\n0.00 0.00 0.01 0.00\r\n0.00 0.01 0.01 0.00\r\n0.00 0.01 0.01 0.00\r\n0.00 -0.00 0.00 0.00\r\n0.01 0.01 0.00 0.00\r\n0.01 0.01 0.01 0.00\r\n0.01 0.00 0.01 0.00\r\n0.01 0.00 0.01 0.00\r\n0.01 0.00 0.01 0.00\r\n0.01 0.01 0.01 0.00\r\n0.01 0.01 0.00 0.00\r\n0.00 0.01 0.01 0.00\r\n0.01 0.01 0.01 0.00\r\n0.00 0.01 0.01 0.00\r\n0.01 0.01 0.01 0.00\r\n0.01 0.01 0.01 0.00\r\n0.01 0.01 0.01 0.00\r\n0.00 0.01 0.01 0.00\r\n0.00 0.01 0.00 0.00\r\n0.00 0.01 0.00 0.00\r\n0.01 0.01 0.01 0.00\r\n0.01 0.01 0.01 0.00\r\n0.01 0.01 0.01 0.00\r\n0.01 0.00 0.00 0.00\r\n0.00 0.00 0.01 0.00\r\n0.01 0.01 0.01 0.00\r\n0.01 0.01 0.00 0.00\r\n0.01 0.00 0.01 0.00\r\n0.01 0.01 0.01 0.00\r\n-0.00 0.01 0.01 0.00\r\n0.01 0.01 0.01 0.00\r\n0.01 0.00 0.01 0.00\r\n0.01 0.01 0.00 0.00\r\n0.01 0.01 0.01 0.00\r\n0.00 0.00 0.00 0.00\r\n0.00 0.00 -0.00 0.00\r\n0.00 0.01 0.01 0.00\r\n0.01 0.01 0.01 0.00\r\n0.01 0.00 0.01 0.00\r\n0.00 0.01 0.01 0.00\r\n0.01 0.01 0.01 0.00\r\n0.01 0.01 0.00 0.00\r\n0.01 0.01 0.01 0.00\r\n0.01 0.01 0.01 0.00\r\n0.01 0.01 0.01 0.00\r\n0.01 0.01 0.01 0.00\r\n0.00 0.01 0.00 0.00\r\n0.01 0.01 0.00 0.00\r\n0.01 0.01 0.01 0.00\r\n0.01 0.01 0.01 0.00\r\n0.00 0.01 0.01 0.00\r\n0.00 0.01 0.00 0.00\r\n0.01 0.01 0.01 0.00\r\n0.00 0.01 0.01 0.00\r\n0.01 0.01 0.00 0.00\r\n0.00 0.01 0.00 0.00\r\n0.01 0.00 0.01 0.00\r\n0.00 0.01 0.01 0.00\r\n0.01 0.01 0.00 0.00\r\n0.00 0.01 0.00 0.00\r\n0.00 0.01 0.01 0.00\r\n0.01 0.01 0.01 0.00\r\n0.01 0.01 0.01 0.00\r\n0.00 0.01 0.00 0.00\r\n0.01 0.01 0.01 0.00\r\n0.01 0.01 0.01 0.00\r\n0.00 0.00 0.00 0.00\r\n0.01 0.01 0.01 0.00\r\n0.01 0.01 0.01 0.00\r\n0.01 0.01 0.01 0.00\r\n0.01 0.01 0.02 0.00\r\n0.01 0.01 0.01 0.00\r\n0.01 0.00 0.01 0.00\r\n0.01 0.00 0.01 0.00\r\n0.01 0.00 0.00 0.00\r\n0.01 0.00 0.00 0.00\r\n0.00 0.01 0.01 0.00\r\n0.01 0.01 0.01 0.00\r\n0.00 0.00 0.00 0.00\r\n0.00 -0.00 0.01 0.00\r\n0.01 0.01 0.01 0.00\r\n0.01 0.00 0.00 0.00\r\n0.01 0.00 0.01 0.00\r\n0.01 0.01 0.01 0.00\r\n0.01 0.01 0.00 0.00\r\n0.01 0.01 0.01 0.00\r\n0.01 0.01 0.01 0.00\r\n0.01 0.01 0.01 0.00\r\n0.00 -0.00 0.00 0.00\r\n0.01 0.01 0.01 0.00\r\n0.01 0.01 0.01 0.00\r\n0.00 0.01 0.00 0.00\r\n0.01 0.01 0.01 0.00\r\n0.01 0.01 0.01 0.00\r\n0.01 0.00 0.01 0.00\r\n0.01 0.01 0.01 0.00\r\n0.01 0.01 0.01 0.00\r\n-0.00 0.00 0.00 0.00\r\n0.00 0.01 0.01 0.00\r\n0.01 0.00 0.01 0.00\r\n0.00 0.00 -0.00 0.00\r\n0.00 0.01 0.01 0.00\r\n0.00 0.01 0.01 0.00\r\n0.01 0.00 0.01 0.00\r\n0.01 0.01 0.01 0.00\r\n0.01 0.00 0.01 0.00\r\n0.00 0.01 0.01 0.00\r\n0.01 0.01 0.01 0.00\r\n0.01 0.01 0.02 0.00\r\n0.00 0.00 0.00 0.00\r\n0.01 0.01 0.01 0.00\r\n0.01 0.01 0.01 0.00\r\n0.01 0.01 0.01 0.00\r\n0.00 0.01 0.01 0.00\r\n0.01 0.01 0.01 0.00\r\n0.01 0.01 0.01 0.00\r\n0.00 0.01 0.00 0.00\r\n0.01 0.00 0.01 0.00\r\n0.00 0.01 0.01 0.00\r\n0.00 0.00 0.00 0.00\r\n0.01 0.01 0.01 0.00\r\n0.01 0.01 0.01 0.00\r\n0.00 0.01 0.00 0.00\r\n0.00 0.00 0.00 0.00\r\n0.01 0.01 0.01 0.00\r\n0.00 0.01 0.01 0.00\r\n0.01 0.01 0.01 0.00\r\n0.01 0.01 0.01 0.00\r\n0.01 0.01 0.01 0.00\r\n0.01 0.01 0.01 0.00\r\n0.01 0.00 -0.00 0.00\r\n0.01 0.00 0.01 0.00\r\n0.01 0.01 0.01 0.00\r\n0.01 0.00 0.01 0.00\r\n0.01 0.01 0.01 0.00\r\n0.01 0.01 0.01 0.00\r\n0.01 0.00 0.00 0.00\r\n0.01 0.01 0.00 0.00\r\n0.00 0.00 0.01 0.00\r\n0.01 0.01 0.00 0.00\r\n0.00 0.00 0.00 0.00\r\n0.01 0.01 0.01 0.00\r\n0.00 0.01 0.00 0.00\r\n0.01 0.01 0.01 0.00\r\n0.01 0.01 0.01 0.00\r\n0.01 0.01 0.01 0.00\r\n0.01 0.00 0.00 0.00\r\n0.00 0.01 0.01 0.00\r\n0.01 0.01 0.01 0.00\r\n0.00 0.00 0.00 0.00\r\n0.01 0.01 0.01 0.00\r\n0.01 0.00 0.00 0.00\r\n0.00 0.01 0.00 0.00\r\n0.01 0.01 0.01 0.00\r\n0.01 0.01 0.00 0.00\r\n0.00 0.01 0.01 0.00\r\n0.00 0.01 0.01 0.00\r\n0.00 0.01 0.00 0.00\r\n0.01 0.01 0.01 0.00\r\n-0.00 0.00 0.00 0.00\r\n0.00 0.00 0.01 0.00\r\n0.00 0.02 0.01 0.00\r\n0.00 0.01 0.00 0.00\r\n0.00 0.00 0.00 0.00\r\n0.01 0.00 0.01 0.00\r\n0.01 0.01 0.00 0.00\r\n0.01 0.01 0.01 0.00\r\n-0.00 0.01 0.00 0.00\r\n0.01 0.01 0.00 0.00\r\n0.01 0.00 0.01 0.00\r\n0.01 0.01 0.01 0.00\r\n0.01 0.01 0.01 0.00\r\n0.01 0.01 0.01 0.00\r\n0.01 0.01 0.01 0.00\r\n0.00 0.02 0.01 0.00\r\n0.01 0.01 0.01 0.00\r\n0.00 0.01 0.00 0.00\r\n0.01 0.01 0.01 0.00\r\n0.01 0.01 0.01 0.00\r\n0.01 0.00 0.00 0.00\r\n0.01 0.01 0.01 0.00\r\n0.01 0.01 0.00 0.00\r\n0.01 0.01 0.01 0.00\r\n0.00 0.01 0.00 0.00\r\n0.01 0.02 0.01 0.00\r\n0.01 0.01 0.01 0.00\r\n0.01 0.01 0.01 0.00\r\n0.01 0.01 0.01 0.00\r\n0.00 0.01 0.01 0.00\r\n0.00 0.01 0.01 0.00\r\n0.01 0.01 0.01 0.00\r\n0.01 0.00 -0.00 0.00\r\n0.00 0.01 0.01 0.00\r\n0.00 0.01 0.01 0.00\r\n0.01 0.01 0.01 0.00\r\n0.01 0.00 0.00 0.00\r\n0.00 0.01 0.00 0.00\r\n0.01 0.01 0.01 0.00\r\n0.01 0.01 0.01 0.00\r\n0.00 0.01 0.01 0.00\r\n0.01 0.01 0.00 0.00\r\n0.01 0.00 0.01 0.00\r\n0.01 0.00 0.01 0.00\r\n0.00 0.01 0.01 0.00\r\n0.01 0.01 0.01 0.00\r\n-0.00 0.01 0.01 0.00\r\n0.01 0.00 0.01 0.00\r\n0.01 0.00 0.01 0.00\r\n0.01 0.01 0.00 0.00\r\n0.01 0.01 0.01 0.00\r\n0.00 -0.00 0.00 0.00\r\n0.00 0.01 0.01 0.00\r\n0.01 0.01 0.01 0.00\r\n0.01 0.01 0.00 0.00\r\n0.01 0.01 0.01 0.00\r\n0.01 0.01 0.01 0.00\r\n0.01 0.01 0.00 0.00\r\n0.01 0.00 0.01 0.00\r\n0.00 0.01 0.00 0.00\r\n-0.00 0.01 0.00 0.00\r\n0.01 0.00 0.01 0.00\r\n0.01 0.01 0.01 0.00\r\n0.00 0.00 0.00 0.00\r\n0.00 0.01 0.01 0.00\r\n0.01 0.01 0.00 0.00\r\n0.01 0.01 0.01 0.00\r\n0.00 0.01 0.01 0.00\r\n0.01 0.00 0.01 0.00\r\n0.01 0.00 0.01 0.00\r\n0.01 0.01 0.01 0.00\r\n0.01 0.01 0.00 0.00\r\n0.01 0.01 0.01 0.00\r\n0.01 0.01 0.00 0.00\r\n0.01 0.01 0.01 0.00\r\n0.01 0.01 0.00 0.00\r\n0.00 0.01 0.01 0.00\r\n0.00 0.01 0.01 0.00\r\n0.01 0.01 0.01 0.00\r\n0.00 0.01 0.01 0.00\r\n0.01 0.01 0.01 0.00\r\n0.01 0.01 0.01 0.00\r\n0.01 0.00 0.01 0.00\r\n0.01 0.01 0.00 0.00\r\n0.01 0.01 0.01 0.00\r\n0.01 0.01 0.01 0.00\r\n0.01 0.01 0.01 0.00\r\n0.00 0.01 0.00 0.00\r\n0.01 0.01 0.01 0.00\r\n0.01 0.01 0.01 0.00\r\n0.01 0.01 0.01 0.00\r\n0.01 0.00 0.01 0.00\r\n0.01 0.01 0.01 0.00\r\n0.01 0.01 0.01 0.00\r\n0.00 0.00 0.00 0.00\r\n0.00 0.01 0.01 0.00\r\n0.01 0.01 0.01 0.00\r\n0.00 0.00 0.00 0.00\r\n0.00 0.00 0.01 0.00\r\n0.01 0.00 0.01 0.00\r\n0.01 0.01 0.00 0.00\r\n0.00 0.01 0.01 0.00\r\n0.01 0.00 0.01 0.00\r\n0.01 0.00 0.01 0.00\r\n0.00 0.01 0.01 0.00\r\n0.01 0.01 0.00 0.00\r\n0.01 0.02 0.01 0.00\r\n0.01 0.00 0.00 0.00\r\n0.01 0.00 0.01 0.00\r\n0.01 0.00 0.01 0.00\r\n0.00 0.01 0.01 0.00\r\n0.01 0.01 0.01 0.00\r\n0.01 0.01 0.01 0.00\r\n0.00 0.01 0.01 0.00\r\n0.01 0.01 0.01 0.00\r\n0.01 0.00 0.01 0.00\r\n0.01 0.01 0.01 0.00\r\n0.01 0.01 0.01 0.00\r\n0.01 0.00 0.00 0.00\r\n0.01 0.00 0.00 0.00\r\n0.01 0.01 0.01 0.00\r\n0.02 0.00 0.01 0.00\r\n0.01 0.01 0.01 0.00\r\n0.01 0.01 0.01 0.00\r\n0.01 0.01 0.01 0.00\r\n0.01 0.00 0.00 0.00\r\n-0.00 0.01 0.01 0.00\r\n0.01 0.01 0.00 0.00\r\n0.01 0.01 0.00 0.00\r\n0.00 0.01 0.01 0.00\r\n0.01 0.00 0.01 0.00\r\n0.01 0.01 0.01 0.00\r\n0.01 0.01 0.01 0.00\r\n0.01 0.00 0.00 0.00\r\n0.01 0.00 0.01 0.00\r\n0.01 0.01 0.00 0.00\r\n0.01 0.01 0.01 0.00\r\n0.00 0.01 0.00 0.00\r\n0.00 0.01 0.01 0.00\r\n0.01 0.00 0.01 0.00\r\n-0.00 0.00 0.01 0.00\r\n-0.00 0.01 0.00 0.00\r\n0.01 0.01 0.01 0.00\r\n0.01 0.01 0.01 0.00\r\n0.00 0.01 0.01 0.00\r\n0.01 0.01 0.01 0.00\r\n0.01 0.01 0.01 0.00\r\n0.00 0.01 0.00 0.00\r\n0.01 0.01 0.01 0.00\r\n0.01 0.00 0.01 0.00\r\n0.00 0.02 0.01 0.00\r\n0.01 0.01 0.01 0.00\r\n0.00 0.01 0.00 0.00\r\n0.01 0.01 0.01 0.00\r\n0.01 0.01 0.01 0.00\r\n0.00 0.01 0.01 0.00\r\n0.01 0.00 0.01 0.00\r\n0.01 0.01 0.00 0.00\r\n0.01 0.01 0.00 0.00\r\n"
  in  "Read":bool
  in  "XON/XOFF Characters":T1={"XON"=enum."DC1", "XOFF"=enum."DC3"}
  in  "Serial Settings":T3={"baud rate"=9600, "data bits"=8, "parity"=enum."None", "stop bits"=10, "flow control"=0} {"flow control" items=["None"=0, "XON/XOFF"=1, "RTS/CTS"=2, "DTR/DSR"=4]; "stop bits" items=["1.0"=10, "1.5"=15, "2.0"=20]; "data bits" min=5 max=8 step=1; "baud rate" items=["75"=75, "110"=110, "134"=134, "150"=150, "300"=300, "600"=600, "1200"=1200, "1800"=1800, "2400"=2400, "4800"=4800, "7200"=7200, "9600"=9600, "14400"=14400, "19200"=19200, "28800"=28800, "38400"=38400, "56000"=56000, "57600"=57600, "115200"=115200, "128000"=128000, "230400"=230400]}
  in  "End Read on Termination Character?":bool=TRUE
  in  "VISA resource name":refnum<visa-resource-name>="COM1"
  # "Overview: Demonstrates the use of the VISA functions to write commands to and read responses from a serial instrument continuously in a loop.\nRequirements: NI-VISA Driver\nInstructions:\n1. Run the VI.\n2. Specify a Command and click the Write button.\n3. Read a Response by clicking the Read button.\n4. Click Stop to stop the VI."
  # "0xA is equivalent to a '\\n' character, which is a line feed."
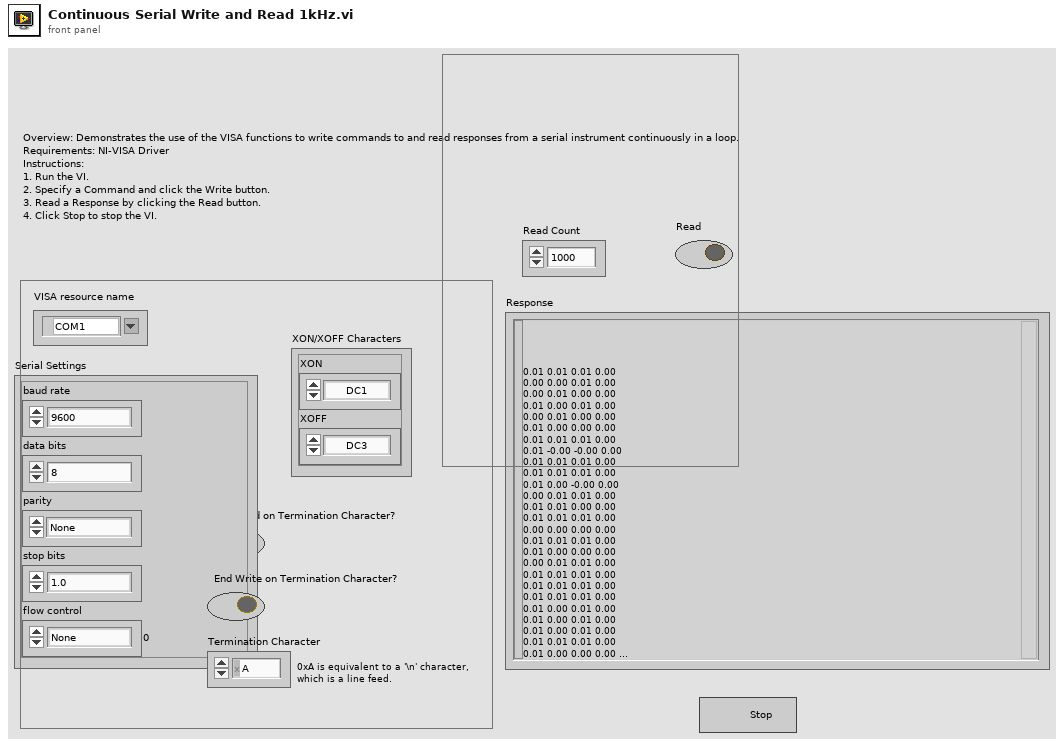
[diagram p1: front panel]
types:
  T1 = typedef "Serial - XON-XOFF Characters.ctl" = cluster{"XON":T2, "XOFF":T2}
  T2 = typedef "Serial - ASCII Characters.ctl" = enum16{"NUL", "SOH", "STX", "ETX", "EOT", "ENQ", "ACK", "BEL", "BS", "HT", "LF", "VT", "FF", "CR", "SO", "SI", "DLE", "DC1", "DC2", "DC3", "DC4", "NAK", "SYN", "ETB", "CAN", "EM", "SUB", "ESC", "FS", "GS", "RS", "US", "SP", "!", "\"", "#", "$", "%", "&", "'", "(", ")", "*", "+", ",", "- (-)", ".", "/", "0", "1", "2", "3", "4", "5", "6", "7", "8", "9", ":", ";", "<", "=", ">", "?", "@", "A", "B", "C", "D", "E", "F", "G", "H", "I", "J", "K", "L", "M", "N", "O", "P", "Q", "R", "S", "T", "U", "V", "W", "X", "Y", "Z", "[", "\\", "]", "^", "_", "`", "a", "b", "c", "d", "e", "f", "g", "h", "i", "j", "k", "l", "m", "n", "o", "p", "q", "r", "s", "t", "u", "v", "w", "x", "y", "z", "{", "|", "}", "~"}
  T3 = typedef "Serial - Settings.ctl" = cluster{"baud rate":u32, "data bits":u16, "parity":enum16{"None", "Odd", "Even", "Mark", "Space"}, "stop bits":u16, "flow control":u16}
  T4 = typedef "XDNodeRunTimeDep.lvlib/timing_clust.ctl" = cluster{"Expected End [f-1]":u64, "Actual End [f-1]":u64, "Finished Late? [f-1]":bool, "Expected End [i-1]":u64, "Actual End [i-1]":u64, "Finished Late? [i-1]":bool, "Expected Start [i]":u64, "Actual Start [i]":u64, "Expected Start [f]":u64, "Actual Start [f]":u64, "Source Name":string, "Structure Name":string, "Period":i64, "Deadline":i64, "Offset":i64, "Start":i64, "Priority":i32, "Timeout":i32, "Mode":T5, "Wakeup Reason":T6, "Error":errorcluster, "Source Type":string, "Secondary Source Type":string, "Global End Time":u64, "Global Start Time":u64, "Frame Duration":u64, "Iteration Duration":u64, "Assigned CPU":i32, "I/O Scan Engine Mode":u32}
  T5 = typedef "XDNodeRunTimeDep.lvlib/nitl_modes.ctl" = enum32{"No Change", "Process missed periods, maintain original phase", "Discard missed periods, maintain original phase", "Process missed periods, ignore original phase", "Discard missed periods, ignore original phase"}
  T6 = typedef "XDNodeRunTimeDep.lvlib/wakeup.ctl" = enum32{"Normal", "Aborted", "Asynchronous wakeup", "Timing source error", "Timed loop error", "Timeout"}
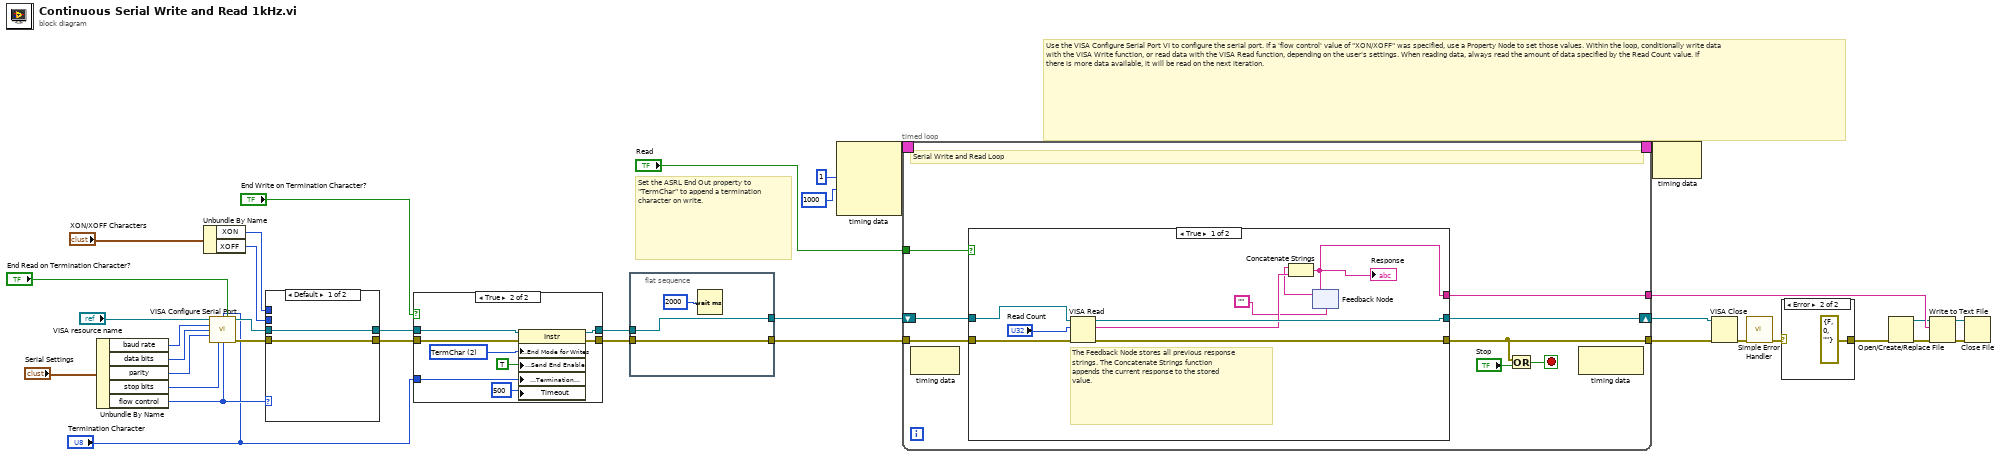
[diagram p0: block diagram]
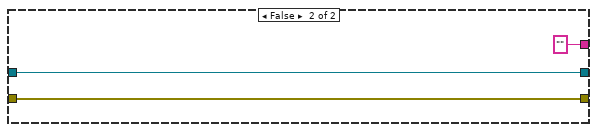
[diagram p3: hidden frame]
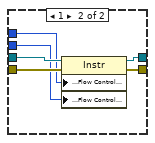
[diagram p5: hidden frame]
diagram:
  # "Set the ASRL End Out property to \"TermChar\" to append a termination character on write."
  # "Use the VISA Configure Serial Port VI to configure the serial port. If a 'flow control' value of \"XON/XOFF\" was specified, use a Property Node to set those values. Within the loop, conditionally write data with the VISA Write function, or read data with the VISA Read function, depending on the user's settings. When reading data, always read the amount of data specified by the Read Count value. If there is more data available, it will be read on the next iteration."
  n1 = Unbundle By Name("Serial Settings") -> ("baud rate"=w29:u32, "data bits"=w30:u16, "parity"=w31:enum16{"None", "Odd", "Even", "Mark", "Space"}, "stop bits"=w32:u16, "flow control"=w24:u16)
  n2 = Unbundle By Name("XON/XOFF Characters") -> ("XON"=w23:T2, "XOFF"=w22:T2)
  n3 = call-poly "VISA Configure Serial Port"("VISA resource name"="VISA resource name", "termination char\n(0xA = '\\n' = LF)"="Termination Character", "Enable Termination\nChar (T)"="End Read on Termination Character?", "baud rate (9600)"=w29, "data bits (8)"=w30, "parity (0:none)"=w31, "stop bits (10: 1 bit)"=w32, "flow control (0:none)"=w24) -> ("VISA resource name out"=w33:refnum<visa-resource-name>, "error out"=w34:errorcluster)  [unwired: 2 in, 4 out]
  n4 = case shown="Default" w24 {
    tunnel: [w37 w44] -> w21
    tunnel: [w38 w43] -> w20
    tunnel: w34 -> [w37 w42]
    tunnel: w33 -> [w38 w41]
    tunnel: w23 -> [_ w40]
    tunnel: w22 -> [_ w39]
    frame Default {
    }
    frame 1 {
      n5 = property class="Instr"(reference=w41, error in=w42, "Serial Settings:Flow Control XON Character"=w40, "Serial Settings:Flow Control XOFF Character"=w39) -> (reference out=w43:refnum<visa-resource-name>, error out=w44:errorcluster)
    }
  }
  n6 = case shown="True" "End Write on Termination Character?" {
    tunnel: w20 -> [w45 w54]
    tunnel: w21 -> [w46 w53]
    tunnel: [w45 w52] -> w1
    tunnel: [w46 w51] -> w3
    tunnel: "Termination Character" -> [_ w49]
    frame False {
    }
    frame True {
      w50 = u16 2 items=["None", "LastBit", "TermChar", "Break"] ("Serial Settings:Serial End Mode for Writes")
      n7 = property class="Instr"(reference=w54, error in=w53, "Serial Settings:End Mode for Writes"=w50, "Message Based Settings:Send End Enable"=TRUE, "Message Based Settings:Termination Character"=w49, "Timeout"=u32 500 ("General Settings:Timeout Value")) -> (reference out=w52:refnum<visa-resource-name>, error out=w51:errorcluster)
    }
  }
  n8 = flat-sequence {
    tunnel: [w55] -> w4
    tunnel: w3 -> [w55]
    tunnel: [w57] -> w2
    tunnel: w1 -> [w57]
    frame #0 {
      n9 = Wait (ms)(milliseconds to wait=u32 2000) -> ()  [unwired: 1 out]
    }
  }
  n10 = node-c288(i64 1 ("Period"), 1000 ("Priority")) -> (w12:T4)  [unwired: 2 in]
  n11 = timed-loop {
    shift-right: [w65] -> w25
    shift-left: w2 -> [w58]
    tunnel: w4 -> [w59]
    tunnel: [w63] -> w26
    tunnel: [w61] -> w17
    timing: w12 -> [_]
    timing-out: [_] -> w11
    tunnel: "Read" -> [w60]
    stop <- w64 stop-if-true
    # "Serial Write and Read Loop"
    n12 = node-c288() -> ()  [unwired: 1 in, 1 out]
    n13 = case shown="True" w60 {
      tunnel: [w74 w79] -> w65
      tunnel: w58 -> [w76 w79]
      tunnel: [w72 w78] -> w63
      tunnel: w59 -> [w75 w78]
      tunnel: [w69 ""] -> w61
      frame True {
        # "The Feedback Node stores all previous response strings. The Concatenate Strings function appends the current response to the stored value."
        n14 = VISA Read(VISA resource name=w76, byte count="Read Count", error in (no error)=w75) -> (VISA resource name out=w74:refnum<visa-resource-name>, read buffer=w71:string, error out=w72:errorcluster)  [unwired: 1 out]
        n15 = feedback #1("") -> (w70:string)
        n16 = Concatenate Strings(w70, w71) -> (w69:string)
        "Response" <- w69
        n17 = feedback-in #1(w69) -> ()
      }
      frame False {
      }
    }
    n18 = Or(x=w63, y="Stop") -> (x .or. y?=w64:bool)
    n19 = node-c288() -> ()  [unwired: 1 in, 1 out]
  }
  n20 = node-c288(w11) -> ()  [unwired: 1 out]
  n21 = VISA Close(VISA resource name=w25, error in (no error)=w26) -> (error out=w6:errorcluster)
  n22 = call <vilib>:"Simple Error Handler.vi"("error in (no error)"=w6) -> ("error out"=w5:errorcluster)  [unwired: 1 in, 7 out]
  n23 = case shown="Error" w5 {
    selector: w5 -> [w80 _]
    tunnel: [w80 errorcluster {"status"=FALSE, "code"=0, "source"=""} ("error constant")] -> w7
    frame No Error {
    }
    frame Error {
    }
  }
  n24 = Open/Create/Replace File(error in=w7) -> (refnum out=w15:refnum<file>, error out=w16:errorcluster)  [unwired: 5 in, 1 out]
  n25 = Write to Text File(file (use dialog)=w15, text=w17, error in=w16) -> (refnum out=w13:refnum<file>, error out=w14:errorcluster)  [unwired: 1 in, 1 out]
  n26 = Close File(refnum=w13, error in=w14) -> ()  [unwired: 2 out]
